vi "Evaporation LABView System.vi"() -> ()   [LabVIEW 2018]
uses:
  <vilib>/Utility/file.llb/Read Delimited Spreadsheet (DBL).vi
  <vilib>/Instr/_visa.llb/VISA Configure Serial Port (Instr).vi
  <instrlib>/JULABO DeviceDriver/JULABO DeviceDriver.lvlib
panel:
  in  "Mixing Time":dbl caption="Mixing Time (HH:MM)" format="%<%H:%M>t"
  out "Update Time":string
  out "Torque [Ncm]":string
  in  "Cent. Duration (MM:SS)":dbl caption="Duration\n(MM:SS)" format="%<%M:%S>t"
  in  "Speed":dbl
  in  "Syrup °Bx by Manual RF":dbl format="%#.1f"
  in  "°Bx DM":dbl caption="Syrup + Additive \n°Bx by Manual RF" format="%#.1f"
  out "Boolean 32":bool
  in  "Mixing RPM":dbl
  out "Boolean 28":bool
  out "Theoretical 5 min. TS":dbl caption="5 min." format="%#.2g"
  out "Boolean 33":bool
  in  "Silverson Duration (MM:SS)":dbl caption="Duration (MM:SS)" format="%<%M:%S>t"
  in  "Speed RPM":dbl
  out "Seeding Julabo SS Temp. [°C]":dbl format="%#.2f"
  out "Seeding Julabo Glass Temp. [°C]":dbl format="%#.2f"
  out "Seeding RPM":dbl format="%#.2f"
  out "Seeding Kss":dbl format="%#.2f"
  out "Seeding Temp. [°C]":dbl format="%#.1f"
  out "Seeding °Bx":dbl format="%#.2f"
  in  "Comments":string
  in  "Loading Delay":timestamp caption="Loading Delay (HH:MM)" format="%<%H:%M>T"
  in  "Additives":string
  in  "Percentage [%]":dbl format="%#_2g"
  in  "pH":dbl format="%#.2g"
  in  "Temp. [°C]":dbl format="%#.2g"
  in  "Sugar Source":string(combo)
  out "Boolean 23":bool
  out "Elapsed Time":dbl format="%.1f"
  out "Seed Time":timestamp format="%<%H:%M:%S>T"
  out "Total Solids (TS)":dbl format="%#.1g"
  in  "Config Tab":T1(tab)
  in  "Condensate Balance":refnum<visa-resource-name>
  in  "Refractometer":refnum<visa-resource-name>
  in  "Vacuubrand Pump":refnum<visa-resource-name>
  in  "Hei-Torque Stirrer":refnum<visa-resource-name>
  in  "Julabo Glass":refnum<visa-resource-name>="COM3"
  in  "Julabo Stainless Steel":refnum<visa-resource-name>="COM3"
  in  "Peristaltic Balance":refnum<visa-resource-name>
  in  "Peristaltic Pump":refnum<visa-resource-name>
  in  "Vacuubrand Pump":bool
  in  "Refractometer":bool
  in  "Condensate Balance":bool
  in  "Julabo Glass":bool
  in  "Hei-Torque Stirrer":bool
  in  "Peristaltic Balance":bool
  in  "Peristaltic Pump":bool
  out "Peristaltic Pump Restart":bool
  out "Hei-Torque Stirrer Restart":bool
  out "Refractometer Restart":bool
  out "Vacuubrand Pump Restart":bool
  out "Condensate Balance Restart":bool
  out "Peristaltic Balance Restart":bool
  out "Julabo Glass Restart":bool
  out "Julabo SS Restart":bool
  in  "Julabo Stainless Steel":bool
  in  "Stop Program":bool
  in  "Start/Stop\nRecording":bool
  out "Process Start":i32
  in  "Experiment Type":string(combo)
  in  "Operator Name":string
  in  "Experiment Name":string
  in  "Time Interval":dbl caption="Time Interval (MM:SS)" format="%<%M:%S>t"
  out "1 min. TS":dbl caption="1 min." format="%#.2g"
  in  "Graphs Tab":T2(tab)
  out "Supersaturation (Kss)":dbl format="%#.2g"
  out "Supersaturation Graph (Kss)":dbl(graph)
  out "Torque [Ncm]":string
  out "Torque Graph":dbl(graph)
  out "Process 2":dbl(graph)
  out "Process":dbl caption="Evaporation Rate [gr/min.]" format="%#.2g"
  out "TS-Mass Graph":cluster{dbl[], dbl[]}(graph) caption="Tank's Solution Weight [gr] vs. Total Solids [%]"
  out "dTS&dBX Graph":cluster{dbl, "Value":dbl}(graph) caption="dTS & dBX Change Rate [gr/min.]"
  in  "Seeds Added":bool
  in  "Add Seeds":bool
  in  "Method":string(combo)
  in  "Seed Type":string
  in  "Amount [gr]":dbl
  in  "Size (um)":string
  out "Theoretical Addition Rate [gr/min]":dbl format="%#.2g"
  in  "Add Syrup":bool
  in  "Syrup Addition [gr]":dbl(slide) scale=0.0..12500.0
  in  "Yield [%]":dbl
  in  "Emptying 2nd\nCycle [gr]":dbl
  in  "Emptying 1st\nCycle [gr]":dbl
  in  "Feed 2nd Cycle [gr]":dbl
  in  "Feed 1st Cycle [gr]":dbl
  out "Boolean 31":bool
  out "Boolean 27":bool
  out "Boolean 30":bool
  out "Boolean 29":bool
  out "Boolean":bool
  out "Peristaltic Pump":bool
  out "RF Pipe":bool
  out "Boolean 19":bool
  in  "Loading 2nd\nCycle [gr]":dbl
  in  "Loading 1st\nCycle [gr]":dbl
  out "Boolean 22":bool
  out "Boolean 2":bool
  out "Vacuubrand Pump":bool
  out "Temp. [°C]":dbl format="%#.2f"
  out "Temp. [°C] by PT100":dbl format="%#.2f"
  out "Tank's Height [cm]":dbl format="%#.1f"
  out "Tank's\nHeight [cm]":dbl(slide) scale=0.0..70.0
  out "Condensate Weight [gr]":dbl format="%#.1f"
  out "Torque [Ncm]":string
  out "Temp. [°C] by RF":dbl format="%#.1f"
  out "°Bx":dbl format="%#.2f"
  out "Syrup Added [gr]":dbl format="%#.1f"
  out "Addition Rate 1 min. [gr/min]":dbl format="%#.2g"
  in  "Dry Substance [%]":dbl
  in  "Purity (0.92-1.0)":dbl
  out "Total Amount Added [gr]":dbl
  in  "Speed RPM":dbl
  in  "Start/Stop":bool
  out "Syrup Added [gr]":dbl(slide) scale=0.0..12500.0
  out "Dry Substance [%]":dbl(slide) scale=0.0..100.0 scale format="%.2f"
  out "1 min. BX":dbl caption="1 min." format="%#.2g"
  out "Colors4":cluster{u32, u32}[](array[cluster])=[{12369084, 12369084}, {255, 255}, {7995525, 7995525}, {7995525, 7995525}]
  out "Interpolated Data":dbl[][](array[numeric])
  out "Table Value":dbl
  out "Actual Saturation (Kact)":dbl format="%#.2g"
  out "Saturation (Ks)":dbl format="%#.2g"
  in  "°Bx In-Line":dbl caption="°Bx by In-Line RF" format="%#.2f"
  in  "Purity (0.92-1.0)":dbl
  out "5 min.":dbl format="%#.2g"
  out "20 min.":dbl format="%#.2g"
  out "Amount of Dry Substance\n[gr]":dbl
  out "Amount of Sugar [gr]":dbl
  out "Dry Substance [%]":dbl(slide) scale=0.0..100.0 scale format="%.2f"
  out "Sugar [%]":dbl(slide) scale=0.0..100.0 scale format="%.2f"
  out "Refractive Index":dbl format="%#.5f"
  out "Temp. [°C]":dbl format="%#.1f"
  out "°Bx":dbl format="%#.2f"
  out "Stirrer Paddle":bool
  out "Tank's Solution\nWeight [gr]":dbl(slide) scale=0.0..12500.0
  out "Boolean 17":bool
  out "Boolean 16":bool
  out "Boolean 15":bool
  out "Boolean 14":bool
  out "Boolean 13":bool
  out "Boolean 12":bool
  out "Boolean 11":bool
  out "Boolean 10":bool
  out "Condensate Weight [gr]":dbl(slide) scale=0.0..3500.0
  out "Boolean 9":bool
  out "Boolean 8":bool
  out "Boolean 7":bool
  out "Boolean 6":bool
  out "Boolean 5":bool
  out "Boolean 4":bool
  out "Boolean 3":bool
  out "Boolean 1":bool
  out "Internal Temp.":dbl(slide) scale=0.0..150.0
  in  "Start/\nStop":bool
  in  "Set Temp. [°C]":dbl format="%.2f"
  out "Internal Temp.":dbl(slide) scale=0.0..150.0
  in  "Start/\nStop":bool
  in  "Set Temp. [°C]":dbl format="%.2f"
  in  "Set Speed RPM":dbl
  in  "Set Vacuum [mbar]":dbl
  in  "Start/Stop":bool
  in  "Vent":bool
  out "Current\nPressure\n[mbar]":dbl(knob) scale=1050.0..50.0
  out "Boolean 20":bool
  out "Boolean 18":bool
  out "Boolean 21":bool
  out "Boolean 26":bool
  out "Boolean 25":bool
  out "Pipe Delay":dbl
  out "Boolean 24":bool
  # "Amounts Added"
  # "Seeding"
  # "Hei-Torque Stirrer"
  # "Condensate\nBalance"
  # "PT100 Sensor"
  # "Julabo Glass"
  # "Refractometer"
  # "Syrup Loading"
  # "Julabo Stainless Steel"
  # "Silverson Mixer"
  # "Centrifugation"
  # "Syrup Preparation Station"
  # "Peristaltic Pump"
  # "Fluidized Bed Dryer"
  # "Values Updated Every 5 min."
  # "Please make sure\nthat all the\ncentrifugation and\nfluidized bed\ndryer values are\nupdated before\npressing \"Stop\nProgram\" or\n\"Stop Recording\"!"
  # "Evaporation\nRate [gr/min]"
  # "BX Change\nRate [gr/min]"
  # "TS Change\nRate [gr/min]"
  # "Theoretical TS Change\nRate [gr/min]"
  # "Peristaltic Balance"
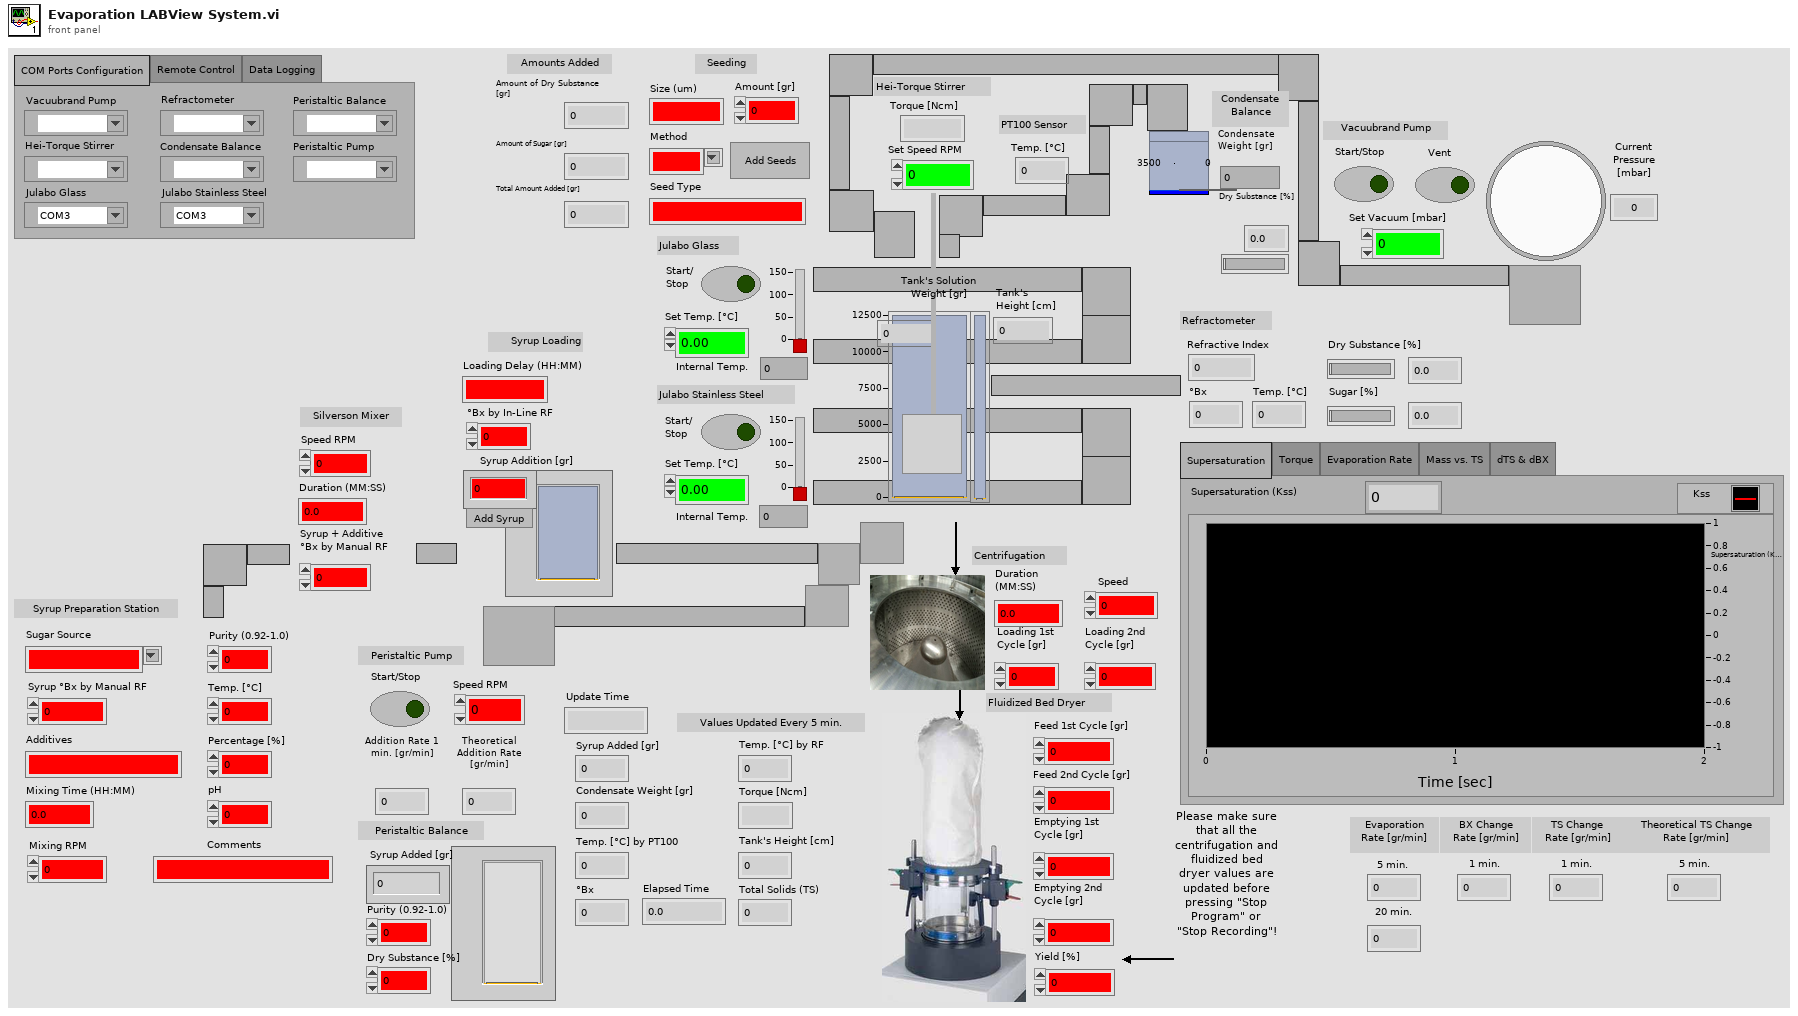
[diagram p1: front panel]
types:
  T1 = enum32{"COM Ports Configuration", "Remote Control", "Data Logging"}
  T2 = enum32{"Supersaturation", "Torque", "Evaporation Rate", "Mass vs. TS", "dTS & dBX"}
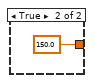
[diagram p5: hidden frame]
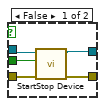
[diagram p6: hidden frame]
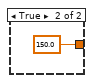
[diagram p10: hidden frame]
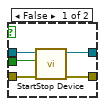
[diagram p11: hidden frame]
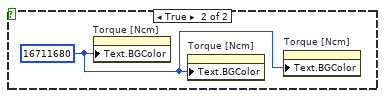
[diagram p16: hidden frame]
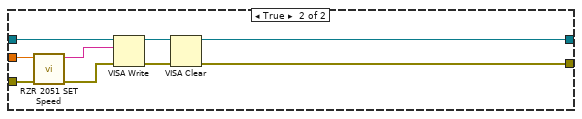
[diagram p17: hidden frame]
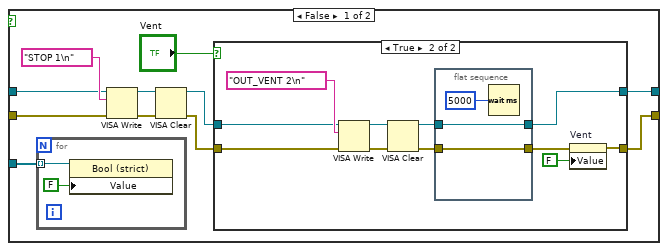
[diagram p20: hidden frame]
diagram:
  n1 = while {
    stop <- w5 stop-if-true
    n2 = property on="Stop Program" class="Bool (strict)"() -> ("Value"=w5:bool)  [unwired: 2 in, 2 out]
    n3 = Wait (ms)(milliseconds to wait=u32 1000) -> ()  [unwired: 1 out]
    n4 = case shown="True" "Vacuubrand Pump" {
      frame False {
      }
      frame True {
        n5 = flat-sequence {
          tunnel: [w26] -> w16
          tunnel: [w25] -> w15
          tunnel: w16 -> [w58]
          tunnel: w15 -> [w57]
          tunnel: [w44] -> w14
          tunnel: [w43] -> w13
          tunnel: [w31] -> w10
          tunnel: w14 -> [w68]
          tunnel: w13 -> [w67]
          tunnel: [w66] -> w12
          tunnel: [w65] -> w11
          tunnel: w10 -> [w64]
          tunnel: [w63] -> w9
          tunnel: w12 -> [w171]
          tunnel: w11 -> [w170]
          tunnel: w9 -> [w160]
          tunnel: [w159] -> w8
          tunnel: [w158] -> w7
          tunnel: w8 -> [w184]
          tunnel: w7 -> [w183]
          frame #0 {
            w27 = u16 10 items=["1.0"=10, "1.5"=15, "2.0"=20] ("stop bits (10: 1 bit)")
            n6 = property on="Start/Stop" class="Bool (strict)"("Value"=FALSE ("PressON/OFF")) -> ()  [unwired: 2 in, 2 out]
            n7 = property on="Vent" class="Bool (strict)"("Value"=FALSE ("PressON/OFF")) -> ()  [unwired: 2 in, 2 out]
            n8 = call-poly "VISA Configure Serial Port"("VISA resource name"="Vacuubrand Pump", "baud rate (9600)"=u32 19200, "data bits (8)"=u16 8, "parity (0:none)"=enum16{"None", "Odd", "Even", "Mark", "Space"}."None", "stop bits (10: 1 bit)"=w27, "flow control (0:none)"=enum16{"None", "XON/XOFF", "RTS/CTS", "DTR/DSR"}."RTS/CTS" ("parity (0:none)")) -> ("VISA resource name out"=w26:refnum<visa-resource-name>, "error out"=w25:errorcluster)  [unwired: 8 in]
            n9 = property on="Set Vacuum [mbar]" class="DigNum (strict)"("Value"=1050.0, "NumText.BGColor"=u32 16711680 ("Numeric Text.Text Colors:BG Color")) -> ()  [unwired: 2 in, 2 out]
            n10 = property on="Current\nPressure\n[mbar]" class="Knob (strict)"("Value"=1050.0 ("Current Pressure [mbar]")) -> ()  [unwired: 2 in, 2 out]
            n11 = property on="Vacuubrand Pump Restart" class="Bool (strict)"("Value"=FALSE ("Vacuubrand Pump Restart")) -> ()  [unwired: 2 in, 2 out]
          }
          frame #1 {
            n12 = control-ref of="Boolean 4"() -> (w37:refnum<vi>)
            n13 = control-ref of="Boolean 3"() -> (w36:refnum<vi>)
            n14 = control-ref of="Boolean 2"() -> (w35:refnum<vi>)
            n15 = control-ref of="Boolean 1"() -> (w34:refnum<vi>)
            n16 = control-ref of="Vacuubrand Pump"() -> (w33:refnum<vi>)
            n17 = VISA Write(VISA resource name=w58, write buffer="REMOTE 1\n" ("Command"), error in (no error)=w57) -> (VISA resource name out=w56:refnum<visa-resource-name>, error out=w55:errorcluster)  [unwired: 1 out]
            n18 = control-ref of="Boolean 9"() -> (w38:refnum<vi>)
            n19 = control-ref of="Boolean 8"() -> (w39:refnum<vi>)
            n20 = control-ref of="Boolean 7"() -> (w40:refnum<vi>)
            n21 = control-ref of="Boolean 6"() -> (w41:refnum<vi>)
            n22 = control-ref of="Boolean 5"() -> (w42:refnum<vi>)
            n23 = VISA Clear(VISA resource name=w56, error in (no error)=w55) -> (VISA resource name out=w54:refnum<visa-resource-name>, error out=w51:errorcluster)
            n24 = VISA Write(VISA resource name=w54, write buffer="CVC 3\n" ("Command"), error in (no error)=w51) -> (VISA resource name out=w53:refnum<visa-resource-name>, error out=w52:errorcluster)  [unwired: 1 out]
            n25 = Build Array(w37, w36, w35, w34, w33, w38, w39, w40, w41, w42) -> (w32:refnum<vi>[])
            n26 = VISA Clear(VISA resource name=w53, error in (no error)=w52) -> (VISA resource name out=w48:refnum<visa-resource-name>, error out=w47:errorcluster)
            n27 = for {
              tunnel: w32 -> [w62] mode=indexing
              tunnel: [w60] -> w31 mode=indexing
              n28 = property class="Bool (strict)"(reference=w62, "Value"=FALSE) -> (reference out=w60:refnum<vi>)  [unwired: 1 in, 1 out]
            }
            n29 = VISA Write(VISA resource name=w48, write buffer="OUT_MODE 2\n" ("Command"), error in (no error)=w47) -> (VISA resource name out=w45:refnum<visa-resource-name>, error out=w46:errorcluster)  [unwired: 1 out]
            n30 = VISA Clear(VISA resource name=w45, error in (no error)=w46) -> (VISA resource name out=w44:refnum<visa-resource-name>, error out=w43:errorcluster)
          }
          frame #2 {
            n31 = while {
              tunnel: w68 -> [w100]
              tunnel: w67 -> [w99]
              shift-right: [w78] -> _
              shift-left: _ -> [w80]
              tunnel: [w94] -> w66
              tunnel: [w93] -> w65
              tunnel: w64 -> [w70]
              tunnel: [w70] -> w63
              stop <- w77 stop-if-true
              n32 = Less?(x="Set Vacuum [mbar]", y=90.0) -> (x < y?=w82:bool)
              n33 = Wait (ms)(milliseconds to wait=u32 1000) -> ()  [unwired: 1 out]
              n34 = case shown="True" w82 {
                tunnel: [w102 90.0] -> w78
                tunnel: "Set Vacuum [mbar]" -> [w102 _]
                frame False {
                }
                frame True {
                  n35 = property on="Set Vacuum [mbar]" class="DigNum (strict)"("Value"=90.0) -> ()  [unwired: 2 in, 2 out]
                }
              }
              n36 = property on="Vacuubrand Pump" class="Bool (strict)"() -> ("Value"=w71:bool)  [unwired: 2 in, 2 out]
              n37 = property on="Stop Program" class="Bool (strict)"() -> ("Value"=w72:bool)  [unwired: 2 in, 2 out]
              n38 = Not(x=w71) -> (.not. x?=w69:bool)
              n39 = Or(x=w69, y=w72) -> (x .or. y?=w77:bool)
              n40 = Not Equal?(x=w78, y=w80) -> (x != y?=w79:bool)
              n41 = case shown="True" w79 {
                tunnel: w78 -> [_ w150]
                tunnel: w99 -> [w147 w155]
                tunnel: w100 -> [w148 w154]
                tunnel: [w148 w153] -> w98
                tunnel: [w147 w152] -> w97
                frame False {
                }
                frame True {
                  n42 = property on="Set Vacuum [mbar]" class="DigNum (strict)"("NumText.BGColor"=u32 65280 ("Numeric Text.Text Colors:BG Color")) -> ()  [unwired: 2 in, 2 out]
                  n43 = call "Crystallization Vaccubrand Pump Set Vacuum.vi"("Vacuum [mbar]"=w150) -> ("DATA OUT"=w151:string)  [unwired: 10 in]
                  n44 = VISA Write(VISA resource name=w154, write buffer=w151, error in (no error)=w155) -> (VISA resource name out=w156:refnum<visa-resource-name>, error out=w157:errorcluster)  [unwired: 1 out]
                  n45 = VISA Clear(VISA resource name=w156, error in (no error)=w157) -> (VISA resource name out=w153:refnum<visa-resource-name>, error out=w152:errorcluster)
                }
              }
              n46 = case shown="True" "Start/Stop" {
                tunnel: w98 -> [w115 w139]
                tunnel: w97 -> [w114 w138]
                tunnel: [w113 w141] -> w96
                tunnel: [w112 w140] -> w95
                tunnel: w70 -> [w108 w137]
                frame False {
                  n47 = for {
                    tunnel: w108 -> [w120] mode=indexing
                    n48 = property class="Bool (strict)"(reference=w120, "Value"=FALSE) -> ()  [unwired: 1 in, 2 out]
                  }
                  n49 = VISA Write(VISA resource name=w115, write buffer="STOP 1\n" ("Command"), error in (no error)=w114) -> (VISA resource name out=w118:refnum<visa-resource-name>, error out=w117:errorcluster)  [unwired: 1 out]
                  n50 = VISA Clear(VISA resource name=w118, error in (no error)=w117) -> (VISA resource name out=w111:refnum<visa-resource-name>, error out=w110:errorcluster)
                  n51 = case shown="True" "Vent" {
                    tunnel: [w122 w128] -> w113
                    tunnel: [w121 w124] -> w112
                    tunnel: w111 -> [w122 w127]
                    tunnel: w110 -> [w121 w126]
                    frame False {
                    }
                    frame True {
                      n52 = VISA Write(VISA resource name=w127, write buffer="OUT_VENT 2\n" ("Command"), error in (no error)=w126) -> (VISA resource name out=w130:refnum<visa-resource-name>, error out=w131:errorcluster)  [unwired: 1 out]
                      n53 = VISA Clear(VISA resource name=w130, error in (no error)=w131) -> (VISA resource name out=w133:refnum<visa-resource-name>, error out=w132:errorcluster)
                      n54 = flat-sequence {
                        tunnel: w133 -> [w136]
                        tunnel: w132 -> [w135]
                        tunnel: [w136] -> w128
                        tunnel: [w135] -> w123
                        frame #0 {
                          n55 = Wait (ms)(milliseconds to wait=u32 5000) -> ()  [unwired: 1 out]
                        }
                      }
                      n56 = property on="Vent" class="Bool (strict)"(error in=w123, "Value"=FALSE ("PressON/OFF")) -> (error out=w124:errorcluster)  [unwired: 1 in, 1 out]
                    }
                  }
                }
                frame True {
                  n57 = for {
                    tunnel: w137 -> [w146] mode=indexing
                    n58 = property class="Bool (strict)"(reference=w146, "Value"=TRUE) -> ()  [unwired: 1 in, 2 out]
                  }
                  n59 = VISA Write(VISA resource name=w139, write buffer="START\n" ("Command"), error in (no error)=w138) -> (VISA resource name out=w144:refnum<visa-resource-name>, error out=w143:errorcluster)  [unwired: 1 out]
                  n60 = VISA Clear(VISA resource name=w144, error in (no error)=w143) -> (VISA resource name out=w141:refnum<visa-resource-name>, error out=w140:errorcluster)
                }
              }
              n61 = VISA Write(VISA resource name=w96, write buffer="IN_PV_1\n" ("Command"), error in (no error)=w95) -> (VISA resource name out=w92:refnum<visa-resource-name>, error out=w91:errorcluster)  [unwired: 1 out]
              n62 = flat-sequence {
                tunnel: w92 -> [w107]
                tunnel: w91 -> [w106]
                tunnel: [w107] -> w90
                tunnel: [w106] -> w89
                frame #0 {
                  n63 = Wait (ms)(milliseconds to wait=u32 500) -> ()  [unwired: 1 out]
                }
              }
              n64 = property class="Instr"(reference=w90, error in=w89) -> (reference out=w88:refnum<visa-resource-name>, error out=w87:errorcluster, "Serial Settings:Number of Bytes at Serial Port"=w86:u32)
              n65 = VISA Read(VISA resource name=w88, byte count=w86, error in (no error)=w87) -> (VISA resource name out=w94:refnum<visa-resource-name>, read buffer=w83:string, error out=w93:errorcluster)  [unwired: 1 out]
              n66 = String Subset(string=w83, length (rest)=4) -> (substring=w74:string)  [unwired: 1 in]
              n67 = Fract/Exp String To Number(string=w74) -> (number=→"Current\nPressure\n[mbar]":dbl)  [unwired: 3 in, 1 out]
            }
          }
          frame #3 {
            n68 = for {
              tunnel: w160 -> [w179] mode=indexing
              n69 = property class="Bool (strict)"(reference=w179, "Value"=FALSE) -> ()  [unwired: 1 in, 2 out]
            }
            n70 = VISA Write(VISA resource name=w171, write buffer="STOP 1\n" ("Command"), error in (no error)=w170) -> (VISA resource name out=w173:refnum<visa-resource-name>, error out=w174:errorcluster)  [unwired: 1 out]
            n71 = VISA Clear(VISA resource name=w173, error in (no error)=w174) -> (VISA resource name out=w168:refnum<visa-resource-name>, error out=w166:errorcluster)
            n72 = VISA Write(VISA resource name=w168, write buffer="OUT_VENT 2\n" ("Command"), error in (no error)=w166) -> (VISA resource name out=w167:refnum<visa-resource-name>, error out=w165:errorcluster)  [unwired: 1 out]
            n73 = VISA Clear(VISA resource name=w167, error in (no error)=w165) -> (VISA resource name out=w164:refnum<visa-resource-name>, error out=w163:errorcluster)
            n74 = flat-sequence {
              tunnel: w164 -> [w182]
              tunnel: w163 -> [w181]
              tunnel: [w182] -> w162
              tunnel: [w181] -> w161
              frame #0 {
                n75 = Wait (ms)(milliseconds to wait=u32 5000) -> ()  [unwired: 1 out]
              }
            }
            n76 = VISA Write(VISA resource name=w162, write buffer="REMOTE 0\n" ("Command"), error in (no error)=w161) -> (VISA resource name out=w176:refnum<visa-resource-name>, error out=w177:errorcluster)  [unwired: 1 out]
            n77 = VISA Clear(VISA resource name=w176, error in (no error)=w177) -> (VISA resource name out=w159:refnum<visa-resource-name>, error out=w158:errorcluster)
          }
          frame #4 {
            n78 = VISA Close(VISA resource name=w184, error in (no error)=w183) -> (error out=w185:errorcluster)
            n79 = call <vilib>:"Simple Error Handler.vi"("error in (no error)"=w185) -> ()  [unwired: 1 in, 8 out]
          }
          frame #5 {
            "Vacuubrand Pump Restart" <- TRUE ("Vacuubrand Pump Restart")
          }
        }
      }
    }
  }
  n80 = while {
    stop <- w187 stop-if-true
    n81 = property on="Stop Program" class="Bool (strict)"() -> ("Value"=w187:bool)  [unwired: 2 in, 2 out]
    n82 = Wait (ms)(milliseconds to wait=u32 1000) -> ()  [unwired: 1 out]
    n83 = case shown="True" "Hei-Torque Stirrer" {
      frame False {
      }
      frame True {
        n84 = flat-sequence {
          tunnel: [w206] -> w198
          tunnel: [w205] -> w199
          tunnel: w199 -> [w213]
          tunnel: w198 -> [w212]
          tunnel: [w215] -> w197
          tunnel: [w214] -> w196
          tunnel: [w211] -> w195
          tunnel: w197 -> [w223]
          tunnel: w196 -> [w220]
          tunnel: w195 -> [w224]
          tunnel: [w225] -> w194
          tunnel: [w222] -> w193
          tunnel: [w221] -> w192
          tunnel: w194 -> [w258]
          tunnel: w193 -> [w260]
          tunnel: w192 -> [w259]
          tunnel: [w262] -> w191
          tunnel: [w261] -> w190
          tunnel: w191 -> [w300]
          tunnel: w190 -> [w301]
          frame #0 {
            w207 = u16 10 items=["1.0"=10, "1.5"=15, "2.0"=20] ("stop bits (10: 1 bit)")
            n85 = property on="Set Speed RPM" class="DigNum (strict)"("Value"=0.0, "NumText.BGColor"=u32 16711680 ("Numeric Text.Text Colors:BG Color")) -> ()  [unwired: 2 in, 2 out]
            n86 = call-poly "VISA Configure Serial Port"("VISA resource name"="Hei-Torque Stirrer", "baud rate (9600)"=u32 9600, "data bits (8)"=u16 8, "parity (0:none)"=enum16{"None", "Odd", "Even", "Mark", "Space"}."None", "stop bits (10: 1 bit)"=w207) -> ("VISA resource name out"=w206:refnum<visa-resource-name>, "error out"=w205:errorcluster)  [unwired: 9 in]
            n87 = property on="Hei-Torque Stirrer Restart" class="Bool (strict)"("Value"=FALSE ("Hei-Torque Stirrer Restart")) -> ()  [unwired: 2 in, 2 out]
            "Stirrer Paddle" <- FALSE ("Stirrer Paddle")
          }
          frame #1 {
            w211 = 0.0 ("Speed RPM")
            # "Start communication to the stirrer"
            n88 = call "RZR 2051 SET Speed.vi"("ERROR IN"=w213, "Speed RPM"=w211) -> ("ERROR OUT"=w217:errorcluster, "DATA OUT"=w216:string)  [unwired: 8 in]
            n89 = VISA Write(VISA resource name=w212, write buffer=w216, error in (no error)=w217) -> (VISA resource name out=w219:refnum<visa-resource-name>, error out=w218:errorcluster)  [unwired: 1 out]
            n90 = VISA Clear(VISA resource name=w219, error in (no error)=w218) -> (VISA resource name out=w214:refnum<visa-resource-name>, error out=w215:errorcluster)
          }
          frame #2 {
            n91 = while {
              tunnel: w223 -> [w240]
              tunnel: [w239] -> w222
              tunnel: [w238] -> w221
              tunnel: w220 -> [w237]
              shift-right: [w233] -> w225
              shift-left: w224 -> [w241]
              stop <- w226 stop-if-true
              n92 = Greater?(x="Set Speed RPM", y=500.0) -> (0:w234:bool)
              n93 = case shown="True" w234 {
                tunnel: [w242 500.0] -> w233
                tunnel: "Set Speed RPM" -> [w242 _]
                frame False {
                }
                frame True {
                  n94 = property on="Set Speed RPM" class="DigNum (strict)"("Value"=500.0) -> ()  [unwired: 2 in, 2 out]
                }
              }
              n95 = Wait (ms)(milliseconds to wait=u32 500) -> ()  [unwired: 1 out]
              n96 = Not Equal?(x=w233, y=w241) -> (x != y?=w227:bool)
              n97 = case shown="True" w227 {
                tunnel: w240 -> [w245 w251]
                tunnel: [w245 w250] -> w239
                tunnel: [w246 w249] -> w238
                tunnel: w237 -> [w246 w248]
                tunnel: w233 -> [_ w247]
                frame False {
                }
                frame True {
                  n98 = call "RZR 2051 SET Speed.vi"("ERROR IN"=w251, "Speed RPM"=w247) -> ("ERROR OUT"=w254:errorcluster, "DATA OUT"=w252:string)  [unwired: 8 in]
                  n99 = VISA Write(VISA resource name=w248, write buffer=w252, error in (no error)=w254) -> (VISA resource name out=w255:refnum<visa-resource-name>, error out=w253:errorcluster)  [unwired: 1 out]
                  n100 = VISA Clear(VISA resource name=w255, error in (no error)=w253) -> (VISA resource name out=w249:refnum<visa-resource-name>, error out=w250:errorcluster)
                }
              }
              n101 = property on="Hei-Torque Stirrer" class="Bool (strict)"() -> ("Value"=w230:bool)  [unwired: 2 in, 2 out]
              n102 = property on="Stop Program" class="Bool (strict)"() -> ("Value"=w231:bool)  [unwired: 2 in, 2 out]
              n103 = Not(x=w230) -> (.not. x?=w229:bool)
              n104 = Or(x=w229, y=w231) -> (x .or. y?=w228:bool)
              n105 = Or(x=w227, y=w228) -> (x .or. y?=w226:bool)
            }
          }
          frame #3 {
            n106 = while {
              tunnel: w260 -> [w276]
              tunnel: w259 -> [w271]
              shift-right: [w268] -> _
              shift-left: w258 -> [w274]
              tunnel: [w273] -> w262
              tunnel: [w272] -> w261
              stop <- w267 stop-if-true
              n107 = property on="Set Speed RPM" class="DigNum (strict)"() -> ("Value"=w265:dbl)  [unwired: 2 in, 2 out]
              n108 = property on="Hei-Torque Stirrer" class="Bool (strict)"() -> ("Value"=w264:bool)  [unwired: 2 in, 2 out]
              n109 = property on="Stop Program" class="Bool (strict)"() -> ("Value"=w266:bool)  [unwired: 2 in, 2 out]
              n110 = Not(x=w264) -> (.not. x?=w263:bool)
              n111 = Greater?(x=w265, y=500.0) -> (0:w270:bool)
              n112 = case shown="True" w270 {
                tunnel: [w278 500.0] -> w268
                tunnel: w265 -> [w278 _]
                frame False {
                }
                frame True {
                  n113 = property on="Set Speed RPM" class="DigNum (strict)"("Value"=500.0) -> ()  [unwired: 2 in, 2 out]
                }
              }
              n114 = Or(x=w263, y=w266) -> (x .or. y?=w267:bool)
              n115 = Wait (ms)(milliseconds to wait=u32 1000) -> ()  [unwired: 1 out]
              n116 = Not Equal?(x=w268, y=w274) -> (x != y?=w275:bool)
              n117 = case shown="False" w275 {
                tunnel: w276 -> [w287 w298]
                tunnel: w271 -> [w285 w297]
                tunnel: [w286 w292] -> w273
                tunnel: [w285 w291] -> w272
                tunnel: w268 -> [_ w290]
                frame False {
                  n118 = call "RZR 2051 Read TORQUE.vi"("ERROR IN"=w287, "COM PORT IN"=w285) -> ("ERROR OUT"=w286:errorcluster, "DATA OUT"=w282:dbl, "STRING OUT"=→"Torque [Ncm]" →"Torque [Ncm]":string)  [unwired: 7 in]
                  "Torque Graph" <- w282
                  n119 = Greater Or Equal?(x=w282, y=50.0) -> (x >= y?=w283:bool)
                  n120 = case shown="False" w283 {
                    frame False {
                      w288 = u32 13816530
                      n121 = property on="Torque [Ncm]" class="Str"("Text.BGColor"=w288) -> ()  [unwired: 2 in, 2 out]
                      n122 = property on="Torque [Ncm]" class="Str"("Text.BGColor"=w288) -> ()  [unwired: 2 in, 2 out]
                      n123 = property on="Torque [Ncm]" class="Str"("Text.BGColor"=w288) -> ()  [unwired: 2 in, 2 out]
                    }
                    frame True {
                      w289 = u32 16711680 ("Numeric Text.Text Colors:BG Color")
                      n124 = property on="Torque [Ncm]" class="Str"("Text.BGColor"=w289) -> ()  [unwired: 2 in, 2 out]
                      n125 = property on="Torque [Ncm]" class="Str"("Text.BGColor"=w289) -> ()  [unwired: 2 in, 2 out]
                      n126 = property on="Torque [Ncm]" class="Str"("Text.BGColor"=w289) -> ()  [unwired: 2 in, 2 out]
                    }
                  }
                }
                frame True {
                  n127 = call "RZR 2051 SET Speed.vi"("ERROR IN"=w298, "Speed RPM"=w290) -> ("ERROR OUT"=w295:errorcluster, "DATA OUT"=w293:string)  [unwired: 8 in]
                  n128 = VISA Write(VISA resource name=w297, write buffer=w293, error in (no error)=w295) -> (VISA resource name out=w296:refnum<visa-resource-name>, error out=w294:errorcluster)  [unwired: 1 out]
                  n129 = VISA Clear(VISA resource name=w296, error in (no error)=w294) -> (VISA resource name out=w291:refnum<visa-resource-name>, error out=w292:errorcluster)
                }
              }
            }
            n130 = property on="Stirrer Paddle" class="Bool (strict)"("Value"=TRUE ("Stirrer Paddle")) -> ()  [unwired: 2 in, 2 out]
            n131 = property on="Set Speed RPM" class="DigNum (strict)"("NumText.BGColor"=u32 65280 ("Numeric Text.Text Colors:BG Color")) -> ()  [unwired: 2 in, 2 out]
          }
          frame #4 {
            n132 = call <instrlib>:"RZR 2051 STOP Communication.vi"("Error IN"=w300, "COM Port"=w301) -> ("Error OUT"=w302:errorcluster)  [unwired: 9 in]
            n133 = property on="Stirrer Paddle" class="Bool (strict)"("Value"=FALSE ("Stirrer Paddle")) -> ()  [unwired: 2 in, 2 out]
            n134 = call <vilib>:"General Error Handler.vi"("error in (no error)"=w302) -> ()  [unwired: 10 in, 5 out]
          }
          frame #5 {
            "Hei-Torque Stirrer Restart" <- TRUE ("Hei-Torque Stirrer Restart")
          }
        }
      }
    }
  }
  n135 = while {
    stop <- w304 stop-if-true
    n136 = property on="Stop Program" class="Bool (strict)"() -> ("Value"=w304:bool)  [unwired: 2 in, 2 out]
    n137 = Wait (ms)(milliseconds to wait=u32 1000) -> ()  [unwired: 1 out]
    n138 = case shown="True" "Peristaltic Pump" {
      frame False {
      }
      frame True {
        n139 = flat-sequence {
          tunnel: [w327] -> w312
          tunnel: [w326] -> w311
          tunnel: [w321] -> w310
          tunnel: w312 -> [w342]
          tunnel: w311 -> [w341]
          tunnel: w310 -> [w335]
          tunnel: [w340] -> w309
          tunnel: [w339] -> w308
          tunnel: [w336] -> w307
          tunnel: w309 -> [w403]
          tunnel: w308 -> [w402]
          tunnel: w307 -> [w405]
          frame #0 {
            w328 = u16 10 items=["1.0"=10, "1.5"=15, "2.0"=20] ("stop bits (10: 1 bit)")
            n140 = control-ref of="Peristaltic Pump"() -> (w319:refnum<vi>)
            n141 = control-ref of="Boolean 29"() -> (w320:refnum<vi>)
            n142 = control-ref of="Boolean 26"() -> (w318:refnum<vi>)
            n143 = control-ref of="Boolean 30"() -> (w317:refnum<vi>)
            n144 = control-ref of="Boolean"() -> (w316:refnum<vi>)
            n145 = Build Array(w319, w320, w318, w317, w316) -> (w322:refnum<vi>[])
            n146 = call-poly "VISA Configure Serial Port"("VISA resource name"="Peristaltic Pump", "baud rate (9600)"=u32 9600, "data bits (8)"=u16 8, "parity (0:none)"=enum16{"None", "Odd", "Even", "Mark", "Space"}."None", "stop bits (10: 1 bit)"=w328, "flow control (0:none)"=enum16{"None", "XON/XOFF", "RTS/CTS", "DTR/DSR"}."None" ("parity (0:none)")) -> ("VISA resource name out"=w327:refnum<visa-resource-name>, "error out"=w326:errorcluster)  [unwired: 8 in]
            n147 = for {
              tunnel: w322 -> [w334] mode=indexing
              tunnel: [w332] -> w321 mode=indexing
              n148 = property class="Bool (strict)"(reference=w334, "Value"=FALSE) -> (reference out=w332:refnum<vi>)  [unwired: 1 in, 1 out]
            }
            n149 = property on="Speed RPM" class="DigNum (strict)"("Value"=0.0 ("Speed RPM"), "NumText.BGColor"=u32 16711680 ("Numeric Text.Text Colors:BG Color")) -> ()  [unwired: 2 in, 2 out]
            n150 = property on="Peristaltic Pump Restart" class="Bool (strict)"("Value"=FALSE ("Peristaltic Pump Restart")) -> ()  [unwired: 2 in, 2 out]
            n151 = property on="Start/Stop" class="Bool (strict)"("Value"=FALSE ("Start/Stop")) -> ()  [unwired: 2 in, 2 out]
          }
          frame #1 {
            n152 = while {
              tunnel: w342 -> [w356]
              tunnel: w341 -> [w355]
              shift-right: [w354] -> _
              shift-left: 0.0 ("Speed RPM") -> [w358]
              tunnel: [w351] -> w340
              tunnel: [w350] -> w339
              shift-right: ["Start/Stop"] -> _
              shift-left: FALSE ("Start/Stop") -> [w352]
              tunnel: [w345] -> w336
              tunnel: w335 -> [w346]
              stop <- w363 stop-if-true
              n153 = property on="Peristaltic Pump" class="Bool (strict)"() -> ("Value"=w362:bool)  [unwired: 2 in, 2 out]
              n154 = Greater?(x="Speed RPM", y=120.0) -> (0:w360:bool)
              n155 = case shown="True" w360 {
                tunnel: "Speed RPM" -> [w399 _]
                tunnel: [w399 120.0 ("Speed RPM")] -> w354
                frame False {
                }
                frame True {
                  n156 = property on="Speed RPM" class="DigNum (strict)"("Value"=120.0 ("Speed RPM")) -> ()  [unwired: 2 in, 2 out]
                }
              }
              n157 = Not(x=w362) -> (.not. x?=w343:bool)
              n158 = property on="Stop Program" class="Bool (strict)"() -> ("Value"=w344:bool)  [unwired: 2 in, 2 out]
              n159 = Wait (ms)(milliseconds to wait=u32 1000) -> ()  [unwired: 1 out]
              n160 = Or(x=w343, y=w344) -> (x .or. y?=w363:bool)
              n161 = Not Equal?(x=w354, y=w358) -> (x != y?=w357:bool)
              n162 = case shown="True" w357 {
                tunnel: w356 -> [w389 w397]
                tunnel: w355 -> [w388 w396]
                tunnel: [w389 w394] -> w348
                tunnel: [w388 w393] -> w349
                tunnel: w354 -> [_ w391]
                frame False {
                }
                frame True {
                  n163 = call "Crystallization Peristaltic Pump Set Speed.vi"("Speed RPM"=w391) -> ("DATA OUT"=w392:string)  [unwired: 10 in]
                  n164 = property on="Speed RPM" class="DigNum (strict)"("NumText.BGColor"=u32 65280 ("Numeric Text.Text Colors:BG Color")) -> ()  [unwired: 2 in, 2 out]
                  n165 = VISA Write(VISA resource name=w397, write buffer=w392, error in (no error)=w396) -> (VISA resource name out=w398:refnum<visa-resource-name>, error out=w395:errorcluster)  [unwired: 1 out]
                  n166 = VISA Clear(VISA resource name=w398, error in (no error)=w395) -> (VISA resource name out=w394:refnum<visa-resource-name>, error out=w393:errorcluster)
                }
              }
              n167 = Not Equal?(x="Start/Stop", y=w352) -> (x != y?=w353:bool)
              n168 = case shown="True" w353 {
                tunnel: [w367 w375] -> w351
                tunnel: [w366 w374] -> w350
                tunnel: w349 -> [w366 w372]
                tunnel: w348 -> [w367 w373]
                tunnel: "Start/Stop" -> [_ w370]
                tunnel: w346 -> [w365 w369]
                tunnel: [w365 w368] -> w345
                frame False {
                }
                frame True {
                  n169 = case shown="True" w370 {
                    tunnel: w369 -> [w379 w384]
                    tunnel: [w378 w383] -> w368
                    frame False {
                      n170 = for {
                        tunnel: w379 -> [w382] mode=indexing
                        tunnel: [w380] -> w378 mode=indexing
                        n171 = property class="Bool (strict)"(reference=w382, "Value"=FALSE) -> (reference out=w380:refnum<vi>)  [unwired: 1 in, 1 out]
                      }
                    }
                    frame True {
                      n172 = for {
                        tunnel: w384 -> [w387] mode=indexing
                        tunnel: [w385] -> w383 mode=indexing
                        n173 = property class="Bool (strict)"(reference=w387, "Value"=TRUE) -> (reference out=w385:refnum<vi>)  [unwired: 1 in, 1 out]
                      }
                    }
                  }
                  n174 = VISA Write(VISA resource name=w373, write buffer="TA2!" ("Command"), error in (no error)=w372) -> (VISA resource name out=w377:refnum<visa-resource-name>, error out=w376:errorcluster)  [unwired: 1 out]
                  n175 = VISA Clear(VISA resource name=w377, error in (no error)=w376) -> (VISA resource name out=w375:refnum<visa-resource-name>, error out=w374:errorcluster)
                }
              }
            }
          }
          frame #2 {
            n176 = for {
              tunnel: w405 -> [w407] mode=indexing
              n177 = property class="Bool (strict)"(reference=w407, "Value"=FALSE) -> ()  [unwired: 1 in, 2 out]
            }
            n178 = VISA Close(VISA resource name=w403, error in (no error)=w402) -> (error out=w404:errorcluster)
            n179 = call <vilib>:"Simple Error Handler.vi"("error in (no error)"=w404) -> ()  [unwired: 1 in, 8 out]
          }
          frame #3 {
            "Peristaltic Pump Restart" <- TRUE ("Peristaltic Pump")
          }
        }
      }
    }
  }
  n180 = while {
    stop <- w410 stop-if-true
    n181 = property on="Stop Program" class="Bool (strict)"() -> ("Value"=w410:bool)  [unwired: 2 in, 2 out]
    n182 = Wait (ms)(milliseconds to wait=u32 1000) -> ()  [unwired: 1 out]
    n183 = case shown="True" "Refractometer" {
      frame False {
        n184 = property on="RF Pipe" class="Bool (strict)"("Value"=FALSE ("RF Pipe")) -> ()  [unwired: 2 in, 2 out]
      }
      frame True {
        n185 = flat-sequence {
          tunnel: [w420] -> w416
          tunnel: [w421] -> w415
          tunnel: w416 -> [w431]
          tunnel: w415 -> [w432]
          tunnel: [w430] -> w414
          tunnel: [w429] -> w413
          tunnel: w414 -> [w496]
          tunnel: w413 -> [w495]
          frame #0 {
            w423 = u16 10 items=["1.0"=10, "1.5"=15, "2.0"=20] ("stop bits (10: 1 bit)")
            n186 = property on="1 min. BX" class="DigNum (strict)"("Value"=0.0 ("1 min. BX")) -> ()  [unwired: 2 in, 2 out]
            n187 = property on="Refractometer Restart" class="Bool (strict)"("Value"=FALSE ("Refractometer Restart")) -> ()  [unwired: 2 in, 2 out]
            n188 = call-poly "VISA Configure Serial Port"("VISA resource name"="Refractometer", "baud rate (9600)"=u32 9600, "data bits (8)"=u16 8, "parity (0:none)"=enum16{"None", "Odd", "Even", "Mark", "Space"}."None", "stop bits (10: 1 bit)"=w423, "flow control (0:none)"=enum16{"None", "XON/XOFF", "RTS/CTS", "DTR/DSR"}."None" ("parity (0:none)")) -> ("VISA resource name out"=w421:refnum<visa-resource-name>, "error out"=w420:errorcluster)  [unwired: 8 in]
          }
          frame #1 {
            n189 = while {
              tunnel: w432 -> [w452]
              tunnel: [w455] -> w430
              tunnel: w431 -> [w451]
              tunnel: [w454] -> w429
              shift-right: [w434] -> _
              shift-left: dbl[] [] -> [w435]
              i -> [w436]
              stop <- w450 stop-if-true
              n190 = property on="Refractometer" class="Bool (strict)"() -> ("Value"=w444:bool)  [unwired: 2 in, 2 out]
              n191 = property class="Instr"(reference=w452, error in=w451) -> (reference out=w447:refnum<visa-resource-name>, error out=w446:errorcluster, "Serial Settings:Number of Bytes at Serial Port"=w445:u32)
              n192 = property on="Stop Program" class="Bool (strict)"() -> ("Value"=w443:bool)  [unwired: 2 in, 2 out]
              n193 = Not(x=w444) -> (.not. x?=w442:bool)
              n194 = Or(x=w442, y=w443) -> (x .or. y?=w450:bool)
              n195 = Greater?(x=w445, y=u32 38) -> (0:w449:bool)
              n196 = case shown="True" w449 {
                tunnel: [w467 w494] -> w455
                tunnel: [w465 w493] -> w454
                tunnel: w445 -> [w470 w484]
                tunnel: w447 -> [w468 w483]
                tunnel: w446 -> [w466 w482]
                frame False {
                  n197 = Greater?(x=w470, y=u32 0) -> (0:w469:bool)
                  n198 = case shown="True" w469 {
                    tunnel: w468 -> [w473 w477]
                    tunnel: [w473 w476] -> w467
                    tunnel: w466 -> [w472 w475]
                    tunnel: [w472 w474] -> w465
                    frame False {
                    }
                    frame True {
                      n199 = VISA Clear(VISA resource name=w477, error in (no error)=w475) -> (VISA resource name out=w476:refnum<visa-resource-name>, error out=w474:errorcluster)
                    }
                  }
                }
                frame True {
                  n200 = VISA Read(VISA resource name=w483, byte count=w484, error in (no error)=w482) -> (VISA resource name out=w494:refnum<visa-resource-name>, read buffer=w478:string, error out=w493:errorcluster)  [unwired: 1 out]
                  n201 = String Subset(string=w478, length (rest)=8) -> (substring=w491:string)  [unwired: 1 in]
                  n202 = String Subset(string=w478, offset (0)=12, length (rest)=4) -> (substring=w489:string)
                  n203 = Fract/Exp String To Number(string=w491) -> (number=→"Refractive Index":dbl)  [unwired: 3 in, 1 out]
                  n204 = Fract/Exp String To Number(string=w489) -> (number=→"Temp. [°C]":dbl)  [unwired: 3 in, 1 out]
                  n205 = String Subset(string=w478, offset (0)=22, length (rest)=5) -> (substring=w486:string)
                  n206 = Fract/Exp String To Number(string=w486) -> (number=→"°Bx":dbl)  [unwired: 3 in, 1 out]
                }
              }
              n207 = Wait (ms)(milliseconds to wait=u32 1000) -> ()  [unwired: 1 out]
              n208 = Add(x=w436, y=1) -> (x+y=w438:i32)
              n209 = Greater?(x=w438, y=59) -> (0:w437:bool)
              n210 = property on="°Bx" class="DigNum (strict)"() -> ("Value"=w433:dbl)  [unwired: 2 in, 2 out]
              n211 = Build Array(w433) -> (w441:dbl[])
              n212 = Insert Into Array(array=w435, index=w436, new element=w441) -> (w434:dbl[])
              n213 = case shown="True" w437 {
                tunnel: w434 -> [_ w460]
                tunnel: w436 -> [_ w459]
                frame False {
                }
                frame True {
                  n214 = Subtract(x=w459, y=59) -> (x-y=w464:i32)
                  n215 = Index Array(array=w460, index #1=w459, index #2=w464) -> (element #1=w461:dbl, element #2=w462:dbl)
                  n216 = property on="1 min. TS" class="DigNum (strict)"() -> ("Value"=w456:dbl)  [unwired: 2 in, 2 out]
                  n217 = Subtract(x=w461, y=w462) -> (x-y=w457:dbl)
                  "1 min. BX" <- w457
                  n218 = Bundle("Value"=w456, w457) -> (→"dTS&dBX Graph":cluster{"Value":dbl, dbl})  [unwired: 1 in]
                }
              }
            }
            "RF Pipe" <- TRUE ("Boolean 29")
          }
          frame #2 {
            n219 = VISA Close(VISA resource name=w496, error in (no error)=w495) -> (error out=w498:errorcluster)
            n220 = property on="RF Pipe" class="Bool (strict)"("Value"=FALSE ("RF Pipe")) -> ()  [unwired: 2 in, 2 out]
            n221 = call <vilib>:"Simple Error Handler.vi"("error in (no error)"=w498) -> ()  [unwired: 1 in, 8 out]
          }
          frame #3 {
            "Refractometer Restart" <- TRUE ("Refractometer Restart")
          }
        }
      }
    }
  }
  n222 = while {
    stop <- w502 stop-if-true
    n223 = property on="Stop Program" class="Bool (strict)"() -> ("Value"=w502:bool)  [unwired: 2 in, 2 out]
    n224 = Wait (ms)(milliseconds to wait=u32 200) -> ()  [unwired: 1 out]
    n225 = case shown="True" "Start/Stop\nRecording" {
      frame False {
      }
      frame True {
        n226 = flat-sequence {
          tunnel: [w531] -> w508
          tunnel: [w532] -> w507
          tunnel: [w543] -> w510
          tunnel: [w544] -> w509
          tunnel: w507 -> [w556]
          tunnel: w508 -> [w555]
          tunnel: w510 -> [w567]
          tunnel: [w569] -> w528
          tunnel: w509 -> [w568]
          tunnel: [w570] -> w527
          tunnel: w528 -> [w582]
          tunnel: [w583] -> w526
          tunnel: w527 -> [w581]
          tunnel: [w584] -> w525
          tunnel: w526 -> [w589]
          tunnel: [w588] -> w524
          tunnel: w525 -> [w590]
          tunnel: [w591] -> w523
          tunnel: w524 -> [w602]
          tunnel: [w601] -> w522
          tunnel: w523 -> [w603]
          tunnel: [w604] -> w521
          tunnel: w522 -> [w621]
          tunnel: [w620] -> w520
          tunnel: w521 -> [w622]
          tunnel: [w623] -> w519
          tunnel: w520 -> [w639]
          tunnel: [w641] -> w518
          tunnel: w519 -> [w640]
          tunnel: [w642] -> w517
          tunnel: w518 -> [w654]
          tunnel: [w652] -> w506
          tunnel: w517 -> [w655]
          tunnel: [w653] -> w504
          tunnel: w506 -> [w668]
          tunnel: [w667] -> w505
          tunnel: w504 -> [w670]
          tunnel: [w669] -> w503
          tunnel: w505 -> [w691]
          tunnel: w503 -> [w692]
          tunnel: [w677] -> w514
          tunnel: [w681] -> w513
          tunnel: w514 -> [w707]
          tunnel: w513 -> [w706]
          tunnel: [w705] -> w512
          tunnel: [w704] -> w511
          tunnel: [w723] -> w530
          tunnel: [w722] -> w529
          tunnel: w512 -> [w717]
          tunnel: w511 -> [w716]
          tunnel: w530 -> [w793]
          tunnel: w529 -> [w792]
          tunnel: [w789] -> w516
          tunnel: [w788] -> w515
          tunnel: w516 -> [w821]
          tunnel: w515 -> [w820]
          frame #0 {
            n227 = Open/Create/Replace File(operation (0:open)=4) -> (refnum out=w541:refnum<file>, error out=w540:errorcluster)  [unwired: 5 in, 1 out]
            n228 = Get Date/Time In Seconds() -> (seconds since 1Jan1904=w535:timestamp)
            n229 = Format Into String(format string="%s,%s,%s,%<%d/%m/%Y>T,%s,%s\\n", initial string=w541, error in=w540, "Experiment Type", "Experiment Name", "Date:" ("Command"), w535, "Operator:" ("Command"), "Operator Name") -> (resulting string=w532:refnum<file>, error out=w531:errorcluster)
          }
          frame #1 {
            n230 = Format Into String(format string="%s,%s,%s,%s,%s,,,,%s,%s\\n%s,%s,,,", initial string=w556, error in=w555, "Sugar Source" ("Command"), "Additive Type" ("Command"), "Seeding Method" ("Command"), "Seed Type" ("Command"), "Time Interval (MM:SS)" ("Command"), "Temp. Julabo Steel [°C]" ("Command"), "Temp. Julabo Glass [°C]" ("Command"), "Sugar Source", "Additives") -> (resulting string=w544:refnum<file>, error out=w543:errorcluster)
          }
          frame #2 {
            n231 = property on="Time Interval" class="DigNum (strict)"() -> ("Value"=w565:dbl)  [unwired: 2 in, 2 out]
            n232 = Format Into String(format string="%<%M:%S>t,,,,\\n%s,,,%s,,,\\n%s,%s,%s,%s,%s,%s\\n", initial string=w568, error in=w567, w565, "Syrup Parameters" ("Command"), "Crystallization Parameters" ("Command"), "Parameter" ("Command"), "Unit" ("Command"), "Value" ("Command"), "Parameter" ("Command"), "Unit" ("Command"), "Value" ("Command")) -> (resulting string=w570:refnum<file>, error out=w569:errorcluster)
          }
          frame #3 {
            n233 = property on="Total Amount Added [gr]" class="DigNum (strict)"() -> ("Value"=w571:dbl)  [unwired: 2 in, 2 out]
            n234 = Format Into String(format string="%s,%s,,%s,%s,,\\n%s,%s,,%s,%s,%.1f\\n", initial string=w581, error in=w582, "Total Syrup" ("Command"), "g" ("Command"), "Total Weight" ("Command"), "g" ("Command"), "Additive Amount" ("Command"), "g" ("Command"), "Starting Weight" ("Command"), "g" ("Command"), w571) -> (resulting string=w584:refnum<file>, error out=w583:errorcluster)
          }
          frame #4 {
            n235 = Format Into String(format string="%s,%s,%.2f,%s,%s,,\\n%s,%s,%.1f,%s,%s,,\\n", initial string=w590, error in=w589, "%Additive" ("Command"), "%" ("Command"), "Percentage [%]", "Feeding Weight" ("Command"), "g" ("Command"), "Syrup °Bx by Manual RF" ("Command"), "Brix" ("Command"), "Syrup °Bx by Manual RF", "Weight Ratio" ("Command"), "%" ("Command")) -> (resulting string=w591:refnum<file>, error out=w588:errorcluster)
          }
          frame #5 {
            n236 = Format Into String(format string="%s,%s,,%s,%s,,\\n%s,%s,%.1f,%s,%s,,\\n", initial string=w603, error in=w602, "Purity" ("Command"), "%" ("Command"), "Agitator" ("Command"), "RPM" ("Command"), "Syrup + Additive °Bx by Manual RF" ("Command"), "Brix" ("Command"), "°Bx DM", "Seed Size" ("Command"), "um" ("Command")) -> (resulting string=w604:refnum<file>, error out=w601:errorcluster)
          }
          frame #6 {
            n237 = property on="°Bx In-Line" class="DigNum (strict)"() -> ("Value"=w619:dbl)  [unwired: 2 in, 2 out]
            n238 = Format Into String(format string="%s,%s,%.2f,%s,%s,,\\n%s,%s,%<%H:%M>t,%s,%s,,\\n", initial string=w622, error in=w621, "°BX by In-Line RF" ("Command"), "Brix" ("Command"), w619, "Seeding Temp." ("Command"), "°C" ("Command"), "Mixing Time" ("Command"), "HH:MM" ("Command"), "Mixing Time", "Seeding °BX" ("Command"), "Brix" ("Command")) -> (resulting string=w623:refnum<file>, error out=w620:errorcluster)
          }
          frame #7 {
            n239 = Format Into String(format string="%s,%s,%d,%s,%s,,\\n%s,%s,%.1f,%s,%s,,\\n", initial string=w640, error in=w639, "Mixing Speed" ("Command"), "RPM" ("Command"), "Mixing RPM", "Seeding Amount" ("Command"), "g" ("Command"), "Temp." ("Command"), "°C" ("Command"), "Temp. [°C]", "Seeding Supersaturation" ("Command"), "NA" ("Command")) -> (resulting string=w642:refnum<file>, error out=w641:errorcluster)
          }
          frame #8 {
            n240 = Format Into String(format string="%s,%s,%.2f,%s,%s,,\\n,,,%s,%s,%<%M:%S>t\\n", initial string=w655, error in=w654, "pH" ("Command"), "NA" ("Command"), "pH", "Seeding Time" ("Command"), "HH:MM:SS" ("Command"), "Silverson Duration" ("Command"), "MM:SS" ("Command"), "Silverson Duration (MM:SS)") -> (resulting string=w653:refnum<file>, error out=w652:errorcluster)
          }
          frame #9 {
            n241 = Format Into String(format string=",,,%s,%s,%d\\n,,,%s,%s,%<%H:%M>T\\n\\n\\n%s,,,,,,,%s,,,,,,,,,,,,,%s\\n", initial string=w670, error in=w668, "Silverson Speed" ("Command"), "RPM" ("Command"), "Speed RPM", "Loading Delay" ("Command"), "HH:MM" ("Command"), "Loading Delay", "Material Data" ("Command"), "Equipment" ("Command"), "Comments" ("Command")) -> (resulting string=w669:refnum<file>, error out=w667:errorcluster)
          }
          frame #10 {
            n242 = Format Into String(format string="%s,%s,%s,%s,%s,%s,%s,%s,%s,%s,,%s,%s,%s,%s,,%s,,%s,%s\\n", initial string=w692, error in=w691, "Time (HH:MM:SS)" ("Command"), "Recording Time [sec]" ("Command"), "Syrup Feed" ("Command"), "Mass Flow" ("Command"), "Water Evaporation" ("Command"), "Evaporation Rate" ("Command"), "Total Mass" ("Command"), "Vacuum" ("Command"), "PT-100" ("Command"), "Refractometer" ("Command"), "Torque" ("Command"), "Pump" ("Command"), "TS Calculated" ("Command"), "Brix Change" ("Command"), "Supersaturation" ("Command"), "Julabo Stainless Steel" ("Command"), "Julabo Glass" ("Command")) -> (resulting string=w677:refnum<file>, error out=w681:errorcluster)
          }
          frame #11 {
            n243 = Format Into String(format string=",,%s,%s,%s,%s,%s,%s,%s,%s,%s,%s,%s,%s,%s,%s,%s,%s,%s,%s\\n", initial string=w707, error in=w706, "g" ("Command"), "g/Min" ("Command"), "g" ("Command"), "g/Min" ("Command"), "g" ("Command"), "mbar" ("Command"), "Temp. [°C]" ("Command"), "% Brix" ("Command"), "Temp. [°C]" ("Command"), "Ncm" ("Command"), "RPM" ("Command"), "% TS" ("Command"), "% Brix" ("Command"), "% Brix_r" ("Command"), "Ref" ("Command"), "TS" ("Command"), "Temp [°C]" ("Command"), "Temp [°C]" ("Command")) -> (resulting string=w705:refnum<file>, error out=w704:errorcluster)
          }
          frame #12 {
            n244 = while {
              shift-right: [w733] -> w723
              shift-left: w717 -> [w734]
              tunnel: w716 -> [w732]
              tunnel: [w731] -> w722
              shift-right: ["Time Interval"] -> _
              shift-left: 0.0 ("Time Interval") -> [w724]
              shift-right: [w728] -> w719
              shift-left: errorcluster {"status"=FALSE, "code"=0, "source"=""} ("error out") -> [w737]
              shift-right: [w725] -> _
              shift-left: 0.0 -> [w726]
              stop <- w727 stop-if-true
              n245 = call "Elapsed Time2"("Time Target (s)"=w724, "Auto Reset"=TRUE, "error in (no error)"=w737) -> ("Time has Elapsed"=w738:bool, "error out"=w736:errorcluster)  [unwired: 9 in, 6 out]
              n246 = case shown="True" w738 {
                tunnel: [w746 w755] -> w728
                tunnel: w736 -> [w746 w755]
                tunnel: w734 -> [w745 w759]
                tunnel: [w745 w758] -> w733
                tunnel: w732 -> [w744 w757]
                tunnel: [w744 w756] -> w731
                tunnel: w726 -> [w743 w752]
                tunnel: [w743 w753] -> w725
                tunnel: w724 -> [_ w750]
                frame False {
                }
                frame True {
                  n247 = Multiply(x=w752, y=w750) -> (x*y=w751:dbl)
                  n248 = Add(x=1.0, y=w752) -> (x+y=w753:dbl)
                  n249 = property on="Condensate Weight [gr]" class="Slide (strict)"() -> ("Value"=w761:dbl)  [unwired: 2 in, 2 out]
                  n250 = property on="Process" class="DigNum (strict)"() -> ("Value"=w762:dbl)  [unwired: 2 in, 2 out]
                  n251 = property on="Tank's Solution\nWeight [gr]" class="Slide (strict)"() -> ("Value"=w763:dbl)  [unwired: 2 in, 2 out]
                  n252 = property on="°Bx" class="DigNum (strict)"() -> ("Value"=w765:dbl)  [unwired: 2 in, 2 out]
                  n253 = property on="Speed RPM" class="DigNum (strict)"() -> ("Value"=w747:dbl)  [unwired: 2 in, 2 out]
                  n254 = property on="Internal Temp." class="Slide (strict)"() -> ("Value"=w748:dbl)  [unwired: 2 in, 2 out]
                  n255 = property on="Internal Temp." class="Slide (strict)"() -> ("Value"=w749:dbl)  [unwired: 2 in, 2 out]
                  n256 = property on="Temp. [°C]" class="DigNum (strict)"() -> ("Value"=w766:dbl)  [unwired: 2 in, 2 out]
                  n257 = property on="Torque [Ncm]" class="Str"() -> ("Value"=w767:string)  [unwired: 2 in, 2 out]
                  n258 = property on="Current\nPressure\n[mbar]" class="Knob (strict)"() -> ("Value"=w764:dbl)  [unwired: 2 in, 2 out]
                  n259 = Get Date/Time In Seconds() -> (seconds since 1Jan1904=w769:timestamp)
                  n260 = property on="Temp. [°C]" class="DigNum (strict)"() -> ("Value"=w768:dbl)  [unwired: 2 in, 2 out]
                  n261 = Format Into String(format string="%<%H:%M:%S>T,%d,,,%.1f,%.3f,%.1f,%.1f,%.1f,%.2f,%.1f,%s,%d,%.1f,%.1f\\n", initial string=w759, error in=w757, w769, w751, w761, w762, w763, w764, w768, w765, w766, w767, w747, w748, w749) -> (resulting string=w758:refnum<file>, error out=w756:errorcluster)
                }
              }
              n262 = property on="Stop Program" class="Bool (strict)"() -> ("Value"=w742:bool)  [unwired: 2 in, 2 out]
              n263 = property on="Start/Stop\nRecording" class="Bool (strict)"() -> ("Value"=w740:bool)  [unwired: 2 in, 2 out]
              n264 = Wait (ms)(milliseconds to wait=u32 10) -> ()  [unwired: 1 out]
              n265 = Not(x=w740) -> (.not. x?=w741:bool)
              n266 = Or(x=w742, y=w741) -> (x .or. y?=w729:bool)
              n267 = Or(x=w728, y=w729) -> (x .or. y?=w727:bool)
            }
            n268 = call <vilib>:"Simple Error Handler.vi"("error in (no error)"=w719) -> ()  [unwired: 4 in, 5 out]
          }
          frame #13 {
            n269 = Format Into String(format string="\\n%s,%s,%s,%s,%s,%s,%s,%s,%s\\n", initial string=w793, error in=w792, "Centrifugation Duration [MM:SS]" ("Command"), "Centrifugation Speed" ("Command"), "Loading 1st Cycle [gr]" ("Command"), "Loading 2nd Cycle [gr]" ("Command"), "Feed 1st Cycle [gr]" ("Command"), "Feed 2nd Cycle [gr]" ("Command"), "Emptying 1st Cycle [gr]" ("Command"), "Emptying 2nd Cycle [gr]" ("Command"), "Yield [%]" ("Command")) -> (resulting string=w795:refnum<file>, error out=w794:errorcluster)
            n270 = Format Into String(format string="%<%M:%S>t,%d,%.2f,%.2f,%.2f,%.2f,%.2f,%.2f,%.2f\\n\\n", initial string=w795, error in=w794, "Cent. Duration (MM:SS)", "Speed", "Loading 1st\nCycle [gr]", "Loading 2nd\nCycle [gr]", "Feed 1st Cycle [gr]", "Feed 2nd Cycle [gr]", "Emptying 1st\nCycle [gr]", "Emptying 2nd\nCycle [gr]", "Yield [%]") -> (resulting string=w789:refnum<file>, error out=w788:errorcluster)
          }
          frame #14 {
            n271 = property on="Seeding Julabo SS Temp. [°C]" class="DigNum (strict)"() -> ("Value"=w804:dbl)  [unwired: 2 in, 2 out]
            n272 = property on="Seeding Julabo Glass Temp. [°C]" class="DigNum (strict)"() -> ("Value"=w803:dbl)  [unwired: 2 in, 2 out]
            n273 = property on="Amount of Sugar [gr]" class="DigNum (strict)"() -> ("Value"=w812:dbl)  [unwired: 2 in, 2 out]
            n274 = property on="Amount of Dry Substance\n[gr]" class="DigNum (strict)"() -> ("Value"=w813:dbl)  [unwired: 2 in, 2 out]
            n275 = property on="Seeding RPM" class="DigNum (strict)"() -> ("Value"=w811:dbl)  [unwired: 2 in, 2 out]
            n276 = property on="Total Amount Added [gr]" class="DigNum (strict)"() -> ("Value"=w814:dbl)  [unwired: 2 in, 2 out]
            n277 = Divide(x=w812, y=w813) -> (x/y=w802:dbl)
            n278 = Multiply(x=w802, y=100.0) -> (x*y=w801:dbl)
            n279 = Format Into String(format string="%s,%.1f,%.1f,%.1f,%.2f,%d,%s,", initial string=w821, error in=w820, "$@!" ("Command"), w804, w803, w814, w801, w811, "Size (um)") -> (resulting string=w819:refnum<file>, error out=w818:errorcluster)
            n280 = property on="Seeding Temp. [°C]" class="DigNum (strict)"() -> ("Value"=w810:dbl)  [unwired: 2 in, 2 out]
            n281 = property on="Seeding °Bx" class="DigNum (strict)"() -> ("Value"=w809:dbl)  [unwired: 2 in, 2 out]
            n282 = property on="Amount [gr]" class="DigNum (strict)"() -> ("Value"=w808:dbl)  [unwired: 2 in, 2 out]
            n283 = property on="Seeding Kss" class="DigNum (strict)"() -> ("Value"=w807:dbl)  [unwired: 2 in, 2 out]
            n284 = property on="Seed Time" class="AbsTime (strict)"() -> ("Value"=w806:timestamp)  [unwired: 2 in, 2 out]
            n285 = property on="Syrup Added [gr]" class="Slide (strict)"() -> ("Value"=w799:dbl)  [unwired: 2 in, 2 out]
            n286 = Format Into String(format string="%.1f,%.2f,%.1f,%.2f,%<%H:%M:%S>T,%.1f,%s,%s\\n", initial string=w819, error in=w818, w810, w809, w808, w807, w806, w799, "Method", "Seed Type") -> (resulting string=w817:refnum<file>)  [unwired: 1 out]
            n287 = Close File(refnum=w817) -> ()  [unwired: 1 in, 2 out]
          }
        }
      }
    }
  }
  n288 = while {
    stop <- w823 stop-if-true
    n289 = property on="Stop Program" class="Bool (strict)"() -> ("Value"=w823:bool)  [unwired: 2 in, 2 out]
    n290 = Wait (ms)(milliseconds to wait=u32 1000) -> ()  [unwired: 1 out]
    n291 = case shown="True" "Condensate Balance" {
      frame False {
      }
      frame True {
        n292 = flat-sequence {
          tunnel: [w853] -> w830
          tunnel: [w854] -> w829
          tunnel: [w843] -> w828
          tunnel: w830 -> [w862]
          tunnel: w829 -> [w861]
          tunnel: w828 -> [w858]
          tunnel: [w864] -> w827
          tunnel: [w863] -> w826
          tunnel: [w858] -> w825
          tunnel: w827 -> [w973]
          tunnel: w826 -> [w972]
          tunnel: w825 -> [w975]
          frame #0 {
            w839 = u16 10 items=["1.0"=10, "1.5"=15, "2.0"=20] ("stop bits (10: 1 bit)")
            n293 = control-ref of="Boolean 17"() -> (w852:refnum<vi>)
            n294 = control-ref of="Boolean 16"() -> (w851:refnum<vi>)
            n295 = control-ref of="Boolean 15"() -> (w850:refnum<vi>)
            n296 = control-ref of="Boolean 14"() -> (w849:refnum<vi>)
            n297 = control-ref of="Boolean 13"() -> (w848:refnum<vi>)
            n298 = control-ref of="Boolean 12"() -> (w847:refnum<vi>)
            n299 = control-ref of="Boolean 11"() -> (w846:refnum<vi>)
            n300 = control-ref of="Boolean 10"() -> (w845:refnum<vi>)
            n301 = Build Array(w852, w851, w850, w849, w848, w847, w846, w845) -> (w844:refnum<vi>[])
            n302 = for {
              tunnel: w844 -> [w857] mode=indexing
              tunnel: [w855] -> w843 mode=indexing
              n303 = property class="Bool (strict)"(reference=w857, "Value"=FALSE) -> (reference out=w855:refnum<vi>)  [unwired: 1 in, 1 out]
            }
            n304 = call-poly "VISA Configure Serial Port"("VISA resource name"="Condensate Balance", "baud rate (9600)"=u32 9600, "data bits (8)"=u16 8, "parity (0:none)"=enum16{"None", "Odd", "Even", "Mark", "Space"}."None", "stop bits (10: 1 bit)"=w839, "flow control (0:none)"=enum16{"None", "XON/XOFF", "RTS/CTS", "DTR/DSR"}."None" ("parity (0:none)")) -> ("VISA resource name out"=w854:refnum<visa-resource-name>, "error out"=w853:errorcluster)  [unwired: 8 in]
            n305 = property on="5 min." class="DigNum (strict)"("Value"=nan ("5 min. acc.")) -> ()  [unwired: 2 in, 2 out]
            n306 = property on="20 min." class="DigNum (strict)"("Value"=nan ("5 min. acc.")) -> ()  [unwired: 2 in, 2 out]
            n307 = property on="Process" class="DigNum (strict)"("Value"=nan ("5 min. acc.")) -> ()  [unwired: 2 in, 2 out]
            n308 = property on="1 min. TS" class="DigNum (strict)"("Value"=nan ("1 min. TS")) -> ()  [unwired: 2 in, 2 out]
            n309 = property on="Theoretical 5 min. TS" class="DigNum (strict)"("Value"=nan ("1 min. TS")) -> ()  [unwired: 2 in, 2 out]
            n310 = property on="Condensate Balance Restart" class="Bool (strict)"("Value"=FALSE ("Condensate Balance Restart")) -> ()  [unwired: 2 in, 2 out]
          }
          frame #1 {
            n311 = while {
              tunnel: [w867] -> w864
              tunnel: [w866] -> w863
              tunnel: w862 -> [w894]
              tunnel: w861 -> [w895]
              shift-right: [w890] -> _
              shift-left: dbl[] [] -> [w888]
              shift-right: [w880] -> _
              shift-left: dbl[] [] -> [w879]
              tunnel: w858 -> [w877]
              i -> [w881]
              stop <- w903 stop-if-true
              n312 = property on="5 min." class="DigNum (strict)"() -> ("Value"=w874:dbl)  [unwired: 2 in, 2 out]
              n313 = Not A Number/Path/Refnum?(number/path/refnum=w874) -> (NaN/Path/Refnum?=w875:bool)
              n314 = Concatenate Strings("Q" ("Command"), "\r", "\n") -> (w899:string)
              n315 = Wait (ms)(milliseconds to wait=u32 200) -> ()  [unwired: 1 out]
              n316 = case shown="True" w875 {
                tunnel: w877 -> [_ w909]
                tunnel: w874 -> [_ w907]
                frame False {
                }
                frame True {
                  n317 = Greater?(x=w907, y=2.0) -> (0:w910:bool)
                  n318 = case shown="True" w910 {
                    tunnel: w909 -> [w911 w915]
                    frame False {
                      n319 = for {
                        tunnel: w911 -> [w914] mode=indexing
                        tunnel: [w912] -> _ mode=indexing
                        n320 = property class="Bool (strict)"(reference=w914, "Value"=FALSE) -> (reference out=w912:refnum<vi>)  [unwired: 1 in, 1 out]
                      }
                    }
                    frame True {
                      n321 = for {
                        tunnel: w915 -> [w918] mode=indexing
                        tunnel: [w916] -> _ mode=indexing
                        n322 = property class="Bool (strict)"(reference=w918, "Value"=TRUE) -> (reference out=w916:refnum<vi>)  [unwired: 1 in, 1 out]
                      }
                    }
                  }
                }
              }
              n323 = VISA Write(VISA resource name=w895, write buffer=w899, error in (no error)=w894) -> (VISA resource name out=w901:refnum<visa-resource-name>, error out=w900:errorcluster)  [unwired: 1 out]
              n324 = property on="Condensate Balance" class="Bool (strict)"() -> ("Value"=w902:bool)  [unwired: 2 in, 2 out]
              n325 = flat-sequence {
                tunnel: w901 -> [w971]
                tunnel: w900 -> [w970]
                tunnel: [w971] -> w869
                tunnel: [w970] -> w868
                frame #0 {
                  n326 = Wait (ms)(milliseconds to wait=u32 100) -> ()  [unwired: 1 out]
                }
              }
              n327 = Not(x=w902) -> (.not. x?=w889:bool)
              n328 = property on="Stop Program" class="Bool (strict)"() -> ("Value"=w904:bool)  [unwired: 2 in, 2 out]
              n329 = Or(x=w889, y=w904) -> (x .or. y?=w903:bool)
              n330 = VISA Read(VISA resource name=w869, byte count=u32 30, error in (no error)=w868) -> (VISA resource name out=w872:refnum<visa-resource-name>, read buffer=w870:string, error out=w871:errorcluster)  [unwired: 1 out]
              n331 = call <instrlib>:"A&D Data Separate.vi"("error in (no error)"=w871, "Received Data"=w870, "VISA resource name"=w872) -> ("error out"=w866:errorcluster, "Value"=w865:dbl, "VISA resource name out"=w867:refnum<visa-resource-name>)  [unwired: 4 in, 2 out]
              "Condensate Weight [gr]" <- w865
              n332 = case shown="True" "Seeds Added" {
                tunnel: w888 -> [_ w932]
                tunnel: w881 -> [_ w931]
                frame False {
                }
                frame True {
                  n333 = property on="Process" class="DigNum (strict)"() -> ("Value"=w933:dbl)  [unwired: 2 in, 2 out]
                  n334 = Not A Number/Path/Refnum?(number/path/refnum=w933) -> (NaN/Path/Refnum?=w934:bool)
                  n335 = case shown="False" w934 {
                    tunnel: w932 -> [w946 _]
                    tunnel: w931 -> [w937 w947]
                    frame False {
                      n336 = Subtract(x=w937, y=1) -> (x-y=w938:i32)
                      n337 = property on="Process Start" class="DigNum (strict)"() -> ("Value"=w936:i32)  [unwired: 2 in, 2 out]
                      n338 = Index Array(array=w946, index #1=w936, index #2=w938) -> (element #1=w941:dbl, element #2=w940:dbl)
                      n339 = Subtract(x=w937, y=w936) -> (x-y=w944:i32)
                      n340 = Subtract(x=w940, y=w941) -> (x-y=w945:dbl)
                      n341 = Divide(x=w944, y=300) -> (x/y=w942:dbl)
                      n342 = Divide(x=w945, y=w942) -> (x/y=→"Process" →"Process 2":dbl)
                    }
                    frame True {
                      n343 = property on="Process" class="DigNum (strict)"("Value"=0.0 ("Process avg.")) -> ()  [unwired: 2 in, 2 out]
                      "Process Start" <- w947
                    }
                  }
                }
              }
              n344 = Build Array(w865) -> (w876:dbl[])
              n345 = Add(x=w881, y=1) -> (x+y=w884:i32)
              n346 = Insert Into Array(array=w888, index=w881, new element=w876) -> (w890:dbl[])
              n347 = Greater?(x=w884, y=299) -> (0:w883:bool)
              n348 = Add(x=w881, y=1) -> (x+y=w891:i32)
              n349 = Greater?(x=w891, y=1499) -> (0:w892:bool)
              n350 = property on="Dry Substance [%]" class="Slide (strict)"() -> ("Value"=w882:dbl)  [unwired: 2 in, 2 out]
              n351 = case shown="True" w892 {
                tunnel: w890 -> [_ w952]
                tunnel: w881 -> [_ w953]
                frame False {
                }
                frame True {
                  n352 = Greater?(x=w953, y=5999) -> (0:w954:bool)
                  n353 = Subtract(x=w953, y=1499) -> (x-y=w959:i32)
                  n354 = case shown="True" w954 {
                    tunnel: w953 -> [_ w962]
                    tunnel: w952 -> [_ w961]
                    frame False {
                    }
                    frame True {
                      n355 = Subtract(x=w962, y=5999) -> (x-y=w968:i32)
                      n356 = Index Array(array=w961, index #1=w962, index #2=w968) -> (element #1=w965:dbl, element #2=w966:dbl)
                      n357 = Subtract(x=w965, y=w966) -> (x-y=w964:dbl)
                      n358 = Divide(x=w964, y=20.0) -> (x/y=→"20 min.":dbl)
                    }
                  }
                  n359 = Index Array(array=w952, index #1=w953, index #2=w959) -> (element #1=w956:dbl, element #2=w957:dbl)
                  n360 = Subtract(x=w956, y=w957) -> (x-y=w951:dbl)
                  n361 = Divide(x=w951, y=5.0) -> (x/y=→"5 min.":dbl)
                }
              }
              n362 = Build Array(w882) -> (w887:dbl[])
              n363 = Insert Into Array(array=w879, index=w881, new element=w887) -> (w880:dbl[])
              n364 = case shown="True" w883 {
                tunnel: w880 -> [_ w920]
                tunnel: w881 -> [_ w919]
                frame False {
                }
                frame True {
                  n365 = flat-sequence {
                    tunnel: w920 -> [w923]
                    tunnel: w919 -> [w922]
                    frame #0 {
                      n366 = Subtract(x=w922, y=299) -> (x-y=w927:i32)
                      n367 = Index Array(array=w923, index #1=w922, index #2=w927) -> (element #1=w924:dbl, element #2=w925:dbl)
                      n368 = Subtract(x=w924, y=w925) -> (x-y=→"1 min. TS":dbl)
                    }
                    frame #1 {
                      n369 = property on="1 min. TS" class="DigNum (strict)"() -> ("Value"=w930:dbl)  [unwired: 2 in, 2 out]
                      n370 = Multiply(x=w930, y=5.0) -> (x*y=→"Theoretical 5 min. TS":dbl)
                    }
                  }
                }
              }
            }
          }
          frame #2 {
            n371 = for {
              tunnel: w975 -> [w977] mode=indexing
              n372 = property class="Bool (strict)"(reference=w977, "Value"=FALSE) -> ()  [unwired: 1 in, 2 out]
            }
            n373 = VISA Close(VISA resource name=w973, error in (no error)=w972) -> (error out=w974:errorcluster)
            n374 = call <vilib>:"Simple Error Handler.vi"("error in (no error)"=w974) -> ()  [unwired: 1 in, 8 out]
          }
          frame #3 {
            "Condensate Balance Restart" <- TRUE ("Condensate Balance Restart")
          }
        }
      }
    }
  }
  n375 = while {
    stop <- w980 stop-if-true
    n376 = property on="Stop Program" class="Bool (strict)"() -> ("Value"=w980:bool)  [unwired: 2 in, 2 out]
    n377 = Wait (ms)(milliseconds to wait=u32 1000) -> ()  [unwired: 1 out]
    n378 = case shown="True" "Peristaltic Balance" {
      frame False {
      }
      frame True {
        n379 = flat-sequence {
          tunnel: [w1000] -> w985
          tunnel: [w1001] -> w984
          tunnel: w985 -> [w1005]
          tunnel: w984 -> [w1004]
          tunnel: [w1007] -> w983
          tunnel: [w1006] -> w982
          tunnel: w983 -> [w1096]
          tunnel: w982 -> [w1095]
          frame #0 {
            w996 = u16 10 items=["1.0"=10, "1.5"=15, "2.0"=20] ("stop bits (10: 1 bit)")
            n380 = property on="Dry Substance [%]" class="DigNum (strict)"("Value"=0.0 ("Dry Substance [%]"), "NumText.BGColor"=u32 16711680 ("Numeric Text.Text Colors:BG Color")) -> ()  [unwired: 2 in, 2 out]
            n381 = property on="Purity (0.92-1.0)" class="DigNum (strict)"("Value"=0.0 ("Purity (0.92-1.0)"), "NumText.BGColor"=u32 16711680 ("Numeric Text.Text Colors:BG Color")) -> ()  [unwired: 2 in, 2 out]
            n382 = call-poly "VISA Configure Serial Port"("VISA resource name"="Peristaltic Balance", "baud rate (9600)"=u32 9600, "data bits (8)"=u16 8, "parity (0:none)"=enum16{"None", "Odd", "Even", "Mark", "Space"}."None", "stop bits (10: 1 bit)"=w996, "flow control (0:none)"=enum16{"None", "XON/XOFF", "RTS/CTS", "DTR/DSR"}."None" ("parity (0:none)")) -> ("VISA resource name out"=w1001:refnum<visa-resource-name>, "error out"=w1000:errorcluster)  [unwired: 8 in]
            n383 = property on="Addition Rate 1 min. [gr/min]" class="DigNum (strict)"("Value"=0.0 ("Addition Rate 1 min. [gr/min]")) -> ()  [unwired: 2 in, 2 out]
            n384 = property on="Syrup Added [gr]" class="Slide (strict)"("Value"=0.0 ("Syrup Added [gr]")) -> ()  [unwired: 2 in, 2 out]
            n385 = property on="Peristaltic Balance Restart" class="Bool (strict)"("Value"=FALSE ("Peristaltic Balance Restart")) -> ()  [unwired: 2 in, 2 out]
            n386 = property on="Theoretical Addition Rate [gr/min]" class="DigNum (strict)"("Value"=nan ("5 min. acc.")) -> ()  [unwired: 2 in, 2 out]
          }
          frame #1 {
            n387 = while {
              tunnel: [w1013] -> w1007
              tunnel: [w1012] -> w1006
              tunnel: w1005 -> [w1054]
              tunnel: w1004 -> [w1055]
              shift-right: [w1048] -> _
              shift-left: dbl[] [] -> [w1049]
              shift-right: [w1008] -> _
              shift-left: 0.0 -> [w1009]
              i -> [w1047]
              stop <- w1057 stop-if-true
              n388 = property on="Purity (0.92-1.0)" class="DigNum (strict)"() -> ("Value"=w1034:dbl)  [unwired: 2 in, 2 out]
              n389 = property on="Dry Substance [%]" class="DigNum (strict)"() -> ("Value"=w1031:dbl)  [unwired: 2 in, 2 out]
              n390 = Not Equal?(x=w1034, y=0.0) -> (x != y?=w1033:bool)
              n391 = Not Equal?(x=0.0 ("y"), y=w1031) -> (x != y?=w1026:bool)
              n392 = property on="5 min." class="DigNum (strict)"() -> ("Value"=w1036:dbl)  [unwired: 2 in, 2 out]
              n393 = Divide(x=w1031, y=100.0) -> (x/y=w1027:dbl)
              n394 = case shown="True" w1033 {
                frame False {
                }
                frame True {
                  n395 = property on="Purity (0.92-1.0)" class="DigNum (strict)"("NumText.BGColor"=u32 65280 ("Numeric Text.Text Colors:BG Color")) -> ()  [unwired: 2 in, 2 out]
                }
              }
              n396 = case shown="True" w1026 {
                frame False {
                }
                frame True {
                  n397 = property on="Dry Substance [%]" class="DigNum (strict)"("NumText.BGColor"=u32 65280 ("Numeric Text.Text Colors:BG Color")) -> ()  [unwired: 2 in, 2 out]
                }
              }
              n398 = Not A Number/Path/Refnum?(number/path/refnum=w1036) -> (NaN/Path/Refnum?=w1039:bool)
              n399 = Concatenate Strings("SI" ("Command"), "\r", "\n") -> (w1023:string)
              n400 = Subtract(x=1.0, y=w1027) -> (x-y=w1028:dbl)
              n401 = Not(x=w1039) -> (.not. x?=w1038:bool)
              n402 = VISA Write(VISA resource name=w1055, write buffer=w1023, error in (no error)=w1054) -> (VISA resource name out=w1025:refnum<visa-resource-name>, error out=w1024:errorcluster)  [unwired: 1 out]
              n403 = And(x=w1026, y=w1038) -> (x .and. y?=w1037:bool)
              n404 = flat-sequence {
                tunnel: w1025 -> [w1081]
                tunnel: w1024 -> [w1080]
                tunnel: [w1081] -> w1010
                tunnel: [w1080] -> w1011
                frame #0 {
                  n405 = Wait (ms)(milliseconds to wait=u32 100) -> ()  [unwired: 1 out]
                }
              }
              n406 = case shown="True" w1037 {
                tunnel: w1028 -> [_ w1085]
                tunnel: w1036 -> [_ w1084]
                frame False {
                  n407 = property on="Theoretical Addition Rate [gr/min]" class="DigNum (strict)"("Value"=nan ("5 min. acc.")) -> ()  [unwired: 2 in, 2 out]
                }
                frame True {
                  n408 = Divide(x=w1084, y=w1085) -> (x/y=→"Theoretical Addition Rate [gr/min]":dbl)
                }
              }
              n409 = property class="Instr"(reference=w1010, error in=w1011) -> (reference out=w1017:refnum<visa-resource-name>, error out=w1018:errorcluster, "Serial Settings:Number of Bytes at Serial Port"=w1015:u32)
              n410 = Greater Or Equal?(x=w1015, y=u32 17) -> (x >= y?=w1016:bool)
              n411 = case shown="False" w1016 {
                tunnel: w1015 -> [_ w1076]
                tunnel: w1018 -> [w1061 w1075]
                tunnel: w1017 -> [w1062 w1074]
                tunnel: [w1062 w1070] -> w1013
                tunnel: [w1061 w1069] -> w1012
                tunnel: [w1060 w1064] -> w1008
                tunnel: w1009 -> [w1060 w1063]
                frame False {
                }
                frame True {
                  n412 = VISA Read(VISA resource name=w1074, byte count=w1076, error in (no error)=w1075) -> (VISA resource name out=w1070:refnum<visa-resource-name>, read buffer=w1073:string, error out=w1069:errorcluster)  [unwired: 1 out]
                  n413 = String Subset(string=w1073, offset (0)=9) -> (substring=w1072:string)  [unwired: 1 in]
                  n414 = Fract/Exp String To Number(string=w1072) -> (offset past number=w1068:i32, number=w1065:dbl)  [unwired: 3 in]
                  n415 = Less?(x=0, y=w1068) -> (x < y?=w1066:bool)
                  n416 = case shown="False" w1066 {
                    tunnel: [w1077 w1078] -> w1064
                    tunnel: w1065 -> [_ w1078]
                    tunnel: w1063 -> [w1077 _]
                    frame False {
                    }
                    frame True {
                    }
                  }
                }
              }
              n417 = Add(x=w1047, y=1) -> (x+y=w1044:i32)
              n418 = Quotient & Remainder(x=w1044, y=300) -> (x-y*floor(x/y)=w1042:i32)  [unwired: 1 out]
              n419 = Greater?(x=w1044, y=299) -> (0:w1045:bool)
              n420 = Equal?(x=0, y=w1042) -> (x = y?=w1040:bool)
              n421 = And(x=w1045, y=w1040) -> (x .and. y?=w1046:bool)
              n422 = property on="Peristaltic Balance" class="Bool (strict)"() -> ("Value"=w1056:bool)  [unwired: 2 in, 2 out]
              n423 = Wait (ms)(milliseconds to wait=u32 200) -> ()  [unwired: 1 out]
              n424 = property on="Stop Program" class="Bool (strict)"() -> ("Value"=w1058:bool)  [unwired: 2 in, 2 out]
              n425 = Not(x=w1056) -> (.not. x?=w1053:bool)
              n426 = Or(x=w1053, y=w1058) -> (x .or. y?=w1057:bool)
              n427 = Build Array(w1008) -> (w1052:dbl[])
              n428 = Absolute Value(x=w1008) -> (abs(x)=→"Syrup Added [gr]":dbl)
              n429 = Insert Into Array(array=w1049, index=w1047, new element=w1052) -> (w1048:dbl[])
              n430 = case shown="True" w1046 {
                tunnel: w1048 -> [_ w1090]
                tunnel: w1047 -> [_ w1089]
                frame False {
                }
                frame True {
                  n431 = Subtract(x=w1089, y=299) -> (x-y=w1094:i32)
                  n432 = Index Array(array=w1090, index #1=w1089, index #2=w1094) -> (element #1=w1091:dbl, element #2=w1092:dbl)
                  n433 = Subtract(x=w1091, y=w1092) -> (x-y=→"Addition Rate 1 min. [gr/min]":dbl)
                }
              }
            }
          }
          frame #2 {
            n434 = VISA Close(VISA resource name=w1096, error in (no error)=w1095) -> (error out=w1097:errorcluster)
            n435 = call <vilib>:"Simple Error Handler.vi"("error in (no error)"=w1097) -> ()  [unwired: 1 in, 8 out]
          }
          frame #3 {
            "Peristaltic Balance Restart" <- TRUE ("Peristaltic Balance Restart")
          }
        }
      }
    }
  }
  n436 = while {
    stop <- w1099 stop-if-true
    n437 = property on="Stop Program" class="Bool (strict)"() -> ("Value"=w1099:bool)  [unwired: 2 in, 2 out]
    n438 = Wait (ms)(milliseconds to wait=u32 1000) -> ()  [unwired: 1 out]
    n439 = case shown="True" "Julabo Stainless Steel" {
      frame False {
      }
      frame True {
        n440 = flat-sequence {
          tunnel: [w1111] -> w1106
          tunnel: [w1110] -> w1105
          tunnel: [w1109] -> w1104
          tunnel: w1106 -> [w1141]
          tunnel: w1105 -> [w1140]
          tunnel: w1104 -> [w1139]
          tunnel: [w1138] -> w1103
          tunnel: [w1137] -> w1102
          tunnel: w1103 -> [w1210]
          tunnel: w1102 -> [w1209]
          frame #0 {
            n441 = control-ref of="Boolean 23"() -> (w1113:refnum<vi>)
            n442 = control-ref of="Boolean 24"() -> (w1108:refnum<vi>)
            n443 = control-ref of="Boolean 22"() -> (w1115:refnum<vi>)
            n444 = control-ref of="Boolean 25"() -> (w1116:refnum<vi>)
            n445 = property on="Internal Temp." class="Slide (strict)"("Value"=0.0) -> ()  [unwired: 2 in, 2 out]
            n446 = property on="Julabo SS Restart" class="Bool (strict)"("Value"=FALSE ("Julabo SS Restart")) -> ()  [unwired: 2 in, 2 out]
            n447 = To Unsigned Long Integer(number=4800) -> (unsigned 32bit integer=w1133:u32)
            n448 = To Unsigned Word Integer(number=2) -> (unsigned 16bit integer=w1132:u16)
            n449 = To Unsigned Word Integer(number=7) -> (unsigned 16bit integer=w1126:u16)
            n450 = To Unsigned Word Integer(number=10) -> (unsigned 16bit integer=w1131:u16)
            n451 = To Unsigned Word Integer(number=2) -> (unsigned 16bit integer=w1130:u16)
            n452 = Build Array(w1113, w1108, w1115, w1116) -> (w1117:refnum<vi>[])
            n453 = for {
              tunnel: w1117 -> [w1136] mode=indexing
              tunnel: [w1134] -> w1111 mode=indexing
              n454 = property class="Bool (strict)"(reference=w1136, "Value"=FALSE) -> (reference out=w1134:refnum<vi>)  [unwired: 1 in, 1 out]
            }
            n455 = property on="Start/\nStop" class="Bool (strict)"("Value"=FALSE ("Start/\nStop")) -> ()  [unwired: 2 in, 2 out]
            n456 = Bundle(w1133, w1132, w1126, w1131, w1130) -> (w1129:cluster{u32, u16, u16, u16, u16})  [unwired: 1 in]
            n457 = property on="Set Temp. [°C]" class="DigNum (strict)"("Value"=0.0, "NumText.BGColor"=u32 16711680 ("Numeric Text.Text Colors:BG Color")) -> ()  [unwired: 2 in, 2 out]
            n458 = To Unsigned Long Integer(number=128) -> (unsigned 32bit integer=w1127:u32)
            n459 = call <instrlib>:"Initialize.vi"("RS485-Address (128: RS232)"=w1127, "Serial Configuration"=w1129, "VISA resource name"="Julabo Stainless Steel") -> ("error out"=w1109:errorcluster, "VISA resource name out"=w1110:refnum<visa-resource-name>)  [unwired: 7 in]
          }
          frame #1 {
            n460 = while {
              tunnel: FALSE ("StartStop") -> [w1155]
              tunnel: w1141 -> [w1153]
              tunnel: w1140 -> [w1152]
              tunnel: w1139 -> [w1151]
              tunnel: [w1150] -> w1138
              tunnel: [w1147] -> w1137
              stop <- w1146 stop-if-true
              n461 = Greater?(x="Set Temp. [°C]", y=150.0) -> (0:w1178:bool)
              n462 = Not Equal?(x=w1155, y="Start/\nStop") -> (x != y?=w1166:bool)
              n463 = case shown="False" w1178 {
                tunnel: [w1185 150.0 ("Set Temp.")] -> w1179
                tunnel: "Set Temp. [°C]" -> [w1184 _]
                frame False {
                  n464 = Less?(x=w1184, y=20.0) -> (x < y?=w1187:bool)
                  n465 = case shown="True" w1187 {
                    tunnel: [w1188 20.0 ("y")] -> w1185
                    tunnel: w1184 -> [w1188 _]
                    frame False {
                    }
                    frame True {
                    }
                  }
                }
                frame True {
                }
              }
              n466 = case shown="True" w1166 {
                tunnel: w1151 -> [w1202 w1208]
                tunnel: w1152 -> [w1203 w1207]
                tunnel: [w1201 w1206] -> w1167
                tunnel: [w1200 w1205] -> w1168
                tunnel: "Start/\nStop" -> [w1199 w1204]
                frame False {
                  n467 = call <instrlib>:"StartStop Device.vi"("error in (no error)"=w1202, "Start/Stop (f:Stop)"=w1199, "VISA resource name"=w1203) -> ("error out"=w1201:errorcluster, "VISA resource name out"=w1200:refnum<visa-resource-name>)  [unwired: 7 in]
                }
                frame True {
                  n468 = call <instrlib>:"StartStop Device.vi"("error in (no error)"=w1208, "Start/Stop (f:Stop)"=w1204, "VISA resource name"=w1207) -> ("error out"=w1206:errorcluster, "VISA resource name out"=w1205:refnum<visa-resource-name>)  [unwired: 7 in]
                }
              }
              n469 = call <instrlib>:"Set Setpoint.vi"("Setpointindex (Setpoint1: Default)"=enum16{"Setpoint 1", "Setpoint 2", "Setpoint 3"}."Setpoint 1" ("Setpoint"), "error in (no error)"=w1167, "newSetpoint (20.00°C)"=w1179, "VISA resource name"=w1168) -> ("error out"=w1170:errorcluster, "VISA resource name out"=w1169:refnum<visa-resource-name>)  [unwired: 6 in]
              n470 = property on="Set Temp. [°C]" class="DigNum (strict)"("Value"=w1179) -> ()  [unwired: 2 in, 2 out]
              n471 = Greater?(x="Set Temp. [°C]", y=0.0) -> (0:w1182:bool)
              n472 = call <instrlib>:"Error Handler.vi"("error in (no error)"=w1170, "ClearCommandError (false)"=TRUE, "VISA resource name"=w1169) -> ("error out"=w1165:errorcluster, "VISA resource name out"=w1171:refnum<visa-resource-name>)  [unwired: 5 in, 2 out]
              n473 = case shown="True" w1182 {
                frame False {
                }
                frame True {
                  n474 = property on="Set Temp. [°C]" class="DigNum (strict)"("NumText.BGColor"=u32 65280 ("Numeric Text.Text Colors:BG Color")) -> ()  [unwired: 2 in, 2 out]
                }
              }
              n475 = call <instrlib>:"Get InternalTemp.vi"("error in (no error)"=w1165, "VISA resource name"=w1171) -> ("error out"=w1147:errorcluster, "InternalTemp (out)"=w1180:dbl, "VISA resource name out"=w1150:refnum<visa-resource-name>)  [unwired: 7 in]
              "Internal Temp." <- w1180
              n476 = Subtract(x=150.0, y=w1180) -> (x-y=w1173:dbl)
              n477 = Subtract(x=w1180, y=20.0) -> (x-y=w1174:dbl)
              n478 = Multiply(x=3.1875, y=w1174) -> (x*y=w1175:dbl)
              n479 = Multiply(x=w1173, y=3.1875) -> (x*y=w1176:dbl)
              n480 = call <vilib>:"RGB to Color.vi"("B"=w1176, "G"=u8 0, "R"=w1175) -> ("Color"=w1172:u32)
              n481 = Bundle("Color"=w1172, "Color"=w1172) -> (w1177:cluster{"Color":u32, "Color":u32})  [unwired: 1 in]
              n482 = for {
                tunnel: w1153 -> [w1194] mode=indexing
                tunnel: w1177 -> [w1195]
                n483 = property class="Bool (strict)"(reference=w1194) -> (reference out=w1193:refnum<vi>, "Colors [4]"=→"Colors4":cluster{u32, u32}[])  [unwired: 1 in, 1 out]
                n484 = property on="Colors4" class="Arr (strict)"() -> ("Value"=w1191:cluster{u32, u32}[])  [unwired: 2 in, 2 out]
                n485 = Replace Array Subset(array=w1191, new element=w1195, index=1) -> (w1196:cluster{u32, u32}[])
                n486 = property class="Bool (strict)"(reference=w1193, "Value"=TRUE, "Colors [4]"=w1196) -> ()  [unwired: 1 in, 2 out]
              }
              n487 = property on="Julabo Stainless Steel" class="Bool (strict)"() -> ("Value"=w1145:bool)  [unwired: 2 in, 2 out]
              n488 = property on="Stop Program" class="Bool (strict)"() -> ("Value"=w1144:bool)  [unwired: 2 in, 2 out]
              n489 = Not(x=w1145) -> (.not. x?=w1149:bool)
              n490 = Wait (ms)(milliseconds to wait=u32 1000) -> ()  [unwired: 1 out]
              n491 = Or(x=w1149, y=w1144) -> (x .or. y?=w1148:bool)
              n492 = Or(x=w1148, y=w1147) -> (x .or. y?=w1146:bool)
            }
          }
          frame #2 {
            n493 = call <instrlib>:"Close.vi"("error in (no error)"=w1209, "VISA resource name"=w1210) -> ("error out"=w1211:errorcluster)  [unwired: 9 in]
            n494 = call <vilib>:"Simple Error Handler.vi"("error in (no error)"=w1211) -> ()  [unwired: 4 in, 5 out]
          }
          frame #3 {
            "Julabo SS Restart" <- TRUE ("Julabo SS Restart")
          }
        }
      }
    }
  }
  n495 = flat-sequence {
    tunnel: [w1249] -> w3
    tunnel: w3 -> [w1255]
    frame #0 {
      w1213 = u32 13816530
      n496 = control-ref of="Boolean 33"() -> (w1216:refnum<vi>)
      n497 = control-ref of="Boolean 32"() -> (w1215:refnum<vi>)
      n498 = control-ref of="Boolean 31"() -> (w1228:refnum<vi>)
      n499 = control-ref of="Boolean 27"() -> (w1227:refnum<vi>)
      n500 = control-ref of="Boolean 30"() -> (w1226:refnum<vi>)
      n501 = control-ref of="Boolean"() -> (w1225:refnum<vi>)
      n502 = control-ref of="Boolean 28"() -> (w1224:refnum<vi>)
      n503 = Build Array(w1216, w1215, w1228, w1227, w1226, w1225, w1224) -> (w1229:refnum<vi>[])
      n504 = property on="Seed Time" class="AbsTime (strict)"("Value"=timestamp(0 s since 1904-01-01) ("Seed Time")) -> ()  [unwired: 2 in, 2 out]
      n505 = for {
        tunnel: w1229 -> [w1252] mode=indexing
        tunnel: [w1250] -> w1249 mode=indexing
        n506 = property class="Bool (strict)"(reference=w1252, "Value"=FALSE) -> (reference out=w1250:refnum<vi>)  [unwired: 1 in, 1 out]
      }
      n507 = call-poly <vilib>:"Read Delimited Spreadsheet.vi"("file path (dialog if empty)"=path "C:/Crystallization System/Sucrose Solubility in Impure Sucrose Solutions Bilinear Interpolated Data.txt") -> ("all rows"=→"Interpolated Data":dbl[][])  [unwired: 9 in, 5 out]
      n508 = property on="Torque [Ncm]" class="Str"("Value"="0" ("Torque [Ncm]"), "Text.BGColor"=w1213) -> ()  [unwired: 2 in, 2 out]
      n509 = property on="TS-Mass Graph" class="XYGraph (strict)"("Value"=cluster{dbl[], dbl[]} {[nan, nan, nan, nan, nan, nan, nan, nan, nan, nan, nan, nan, nan, nan, nan, nan, nan, nan, nan, nan, nan, nan, nan, nan, nan, nan, nan, nan, nan, nan, nan, nan, nan, nan, nan, nan, nan, nan, nan, nan, nan, nan, nan, nan, nan, nan, nan, nan, nan, nan, nan, nan, nan, nan, nan, nan, nan, nan, nan, nan, nan, nan, nan, nan, nan, nan, nan, nan, nan, nan, nan, nan, nan, nan, nan, nan, nan], [0.0, 0.0, 0.0, 0.0, 0.0, 0.0, 0.0, 0.0, 0.0, 0.0, 0.0, 0.0, 0.0, 0.0, 0.0, 0.0, 0.0, 0.0, 0.0, 0.0, 0.0, 0.0, 0.0, 0.0, 0.0, 0.0, 0.0, 0.0, 0.0, 0.0, 0.0, 0.0, 0.0, 0.0, 0.0, 0.0, 0.0, 0.0, 0.0, 0.0, 0.0, 0.0, 0.0, 0.0, 0.0, 0.0, 0.0, 0.0, 0.0, 0.0, 0.0, 0.0, 0.0, 0.0, 0.0, 0.0, 0.0, 0.0, 0.0, 0.0, 0.0, 0.0, 0.0, 0.0, 0.0, 0.0, 0.0, 0.0, 0.0, 0.0, 0.0, 0.0, 0.0, 0.0, 0.0, 0.0, 0.0]} ("TS-Mass Graph")) -> ()  [unwired: 2 in, 2 out]
      n510 = property on="Torque [Ncm]" class="Str"("Value"="0" ("Torque [Ncm]"), "Text.BGColor"=w1213) -> ()  [unwired: 2 in, 2 out]
      n511 = property on="Torque [Ncm]" class="Str"("Value"="0" ("Torque [Ncm]"), "Text.BGColor"=w1213) -> ()  [unwired: 2 in, 2 out]
      n512 = property on="dTS&dBX Graph" class="WFChart (strict)"("History Data"=cluster{dbl, "Value":dbl}[] []) -> ()  [unwired: 2 in, 2 out]
      n513 = property on="Supersaturation Graph (Kss)" class="WFChart (strict)"("History Data"=dbl[] []) -> ()  [unwired: 2 in, 2 out]
      n514 = property on="Torque Graph" class="WFChart (strict)"("History Data"=dbl[] []) -> ()  [unwired: 2 in, 2 out]
      n515 = property on="Process 2" class="WFChart (strict)"("History Data"=dbl[] []) -> ()  [unwired: 2 in, 2 out]
      n516 = property on="Elapsed Time" class="DigNum (strict)"("Value"=0.0 ("Elapsed Time")) -> ()  [unwired: 2 in, 2 out]
      n517 = property on="Tank's\nHeight [cm]" class="Slide (strict)"("Value"=0.0 ("Tank's \nVolume [mL]")) -> ()  [unwired: 2 in, 2 out]
      n518 = property on="Tank's Solution\nWeight [gr]" class="Slide (strict)"("Value"=0.0) -> ()  [unwired: 2 in, 2 out]
      n519 = property on="Total Amount Added [gr]" class="DigNum (strict)"("Value"=0.0 ("Amount of Added Syrup [gr]")) -> ()  [unwired: 2 in, 2 out]
      n520 = property on="Amount of Dry Substance\n[gr]" class="DigNum (strict)"("Value"=0.0) -> ()  [unwired: 2 in, 2 out]
      n521 = property on="Amount of Sugar [gr]" class="DigNum (strict)"("Value"=0.0) -> ()  [unwired: 2 in, 2 out]
      n522 = property on="Actual Saturation (Kact)" class="DigNum (strict)"("Value"=0.0) -> ()  [unwired: 2 in, 2 out]
      n523 = property on="Condensate Weight [gr]" class="Slide (strict)"("Value"=0.0) -> ()  [unwired: 2 in, 2 out]
      n524 = property on="°Bx" class="DigNum (strict)"("Value"=0.0) -> ()  [unwired: 2 in, 2 out]
      n525 = property on="Dry Substance [%]" class="Slide (strict)"("Value"=0.0) -> ()  [unwired: 2 in, 2 out]
      n526 = property on="Sugar [%]" class="Slide (strict)"("Value"=0.0) -> ()  [unwired: 2 in, 2 out]
      n527 = property on="Saturation (Ks)" class="DigNum (strict)"("Value"=0.0) -> ()  [unwired: 2 in, 2 out]
      n528 = property on="Supersaturation (Kss)" class="DigNum (strict)"("Value"=0.0) -> ()  [unwired: 2 in, 2 out]
      n529 = property on="Temp. [°C]" class="DigNum (strict)"("Value"=0.0 ("Temp. [°C]")) -> ()  [unwired: 2 in, 2 out]
      n530 = property on="Temp. [°C]" class="DigNum (strict)"("Value"=0.0) -> ()  [unwired: 2 in, 2 out]
      n531 = property on="Table Value" class="DigNum (strict)"("Value"=0.0) -> ()  [unwired: 2 in, 2 out]
    }
    frame #1 {
      n532 = while {
        shift-right: [w1269] -> _
        shift-left: 0.0 -> [w1307]
        shift-right: [w1271] -> _
        shift-left: 0.0 -> [w1306]
        shift-right: [w1270] -> _
        shift-left: 0.0 -> [w1316]
        tunnel: w1255 -> [w1284]
        shift-right: [w1265] -> _
        shift-left: dbl[] [] -> [w1267]
        shift-right: [w1264] -> _
        shift-left: dbl[] [] -> [w1266]
        i -> [w1274]
        stop <- "Stop Program" stop-if-true
        n533 = case shown="True" "Add Syrup" {
          tunnel: w1316 -> [w1407 w1427]
          tunnel: [w1407 w1415] -> w1294
          tunnel: w1307 -> [w1406 w1425]
          tunnel: [w1406 w1424] -> w1296
          tunnel: w1306 -> [w1405 w1422]
          tunnel: [w1405 w1416] -> w1295
          tunnel: w1284 -> [w1404 w1414]
          frame False {
            n534 = property on="Pipe Delay" class="DigNum (strict)"() -> ("Value"=w1398:dbl)  [unwired: 2 in, 2 out]
            n535 = property on="Boolean 31" class="Bool (strict)"() -> ("Value"=w1402:bool)  [unwired: 2 in, 2 out]
            n536 = Add(x=w1398, y=1.0) -> (x+y=w1399:dbl)
            n537 = Greater?(x=w1398, y=5.0) -> (0:w1401:bool)
            n538 = property on="Pipe Delay" class="DigNum (strict)"("Value"=w1399) -> ()  [unwired: 2 in, 2 out]
            n539 = And(x=w1402, y=w1401) -> (x .and. y?=w1397:bool)
            n540 = case shown="False" w1397 {
              tunnel: w1404 -> [_ w1409]
              frame False {
              }
              frame True {
                n541 = for {
                  tunnel: w1409 -> [w1412] mode=indexing
                  tunnel: [w1410] -> _ mode=indexing
                  n542 = property class="Bool (strict)"(reference=w1412, "Value"=FALSE) -> (reference out=w1410:refnum<vi>)  [unwired: 1 in, 1 out]
                }
              }
            }
            n543 = case shown="False" w1397 {
              frame False {
              }
              frame True {
                "Pipe Delay" <- 0.0 ("Pipe Delay")
              }
            }
          }
          frame True {
            n544 = flat-sequence {
              tunnel: w1425 -> [w1434]
              tunnel: [w1433] -> w1426
              tunnel: ["Syrup Addition [gr]"] -> w1423
              tunnel: [w1436] -> w1424
              tunnel: w1426 -> [w1436]
              frame #0 {
                n545 = Add(x=w1434, y="Syrup Addition [gr]") -> (x+y=w1433:dbl)
              }
              frame #1 {
                n546 = property on="Syrup Addition [gr]" class="Slide (strict)"("Value"=0.0) -> ()  [unwired: 2 in, 2 out]
                "Total Amount Added [gr]" <- w1436
              }
            }
            n547 = for {
              tunnel: w1414 -> [w1431] mode=indexing
              tunnel: [w1429] -> _ mode=indexing
              n548 = property class="Bool (strict)"(reference=w1431, "Value"=TRUE) -> (reference out=w1429:refnum<vi>)  [unwired: 1 in, 1 out]
            }
            n549 = Divide(x="°Bx In-Line", y=100.0) -> (x/y=w1419:dbl)
            n550 = Multiply(x=w1423, y=w1419) -> (x*y=w1421:dbl)
            n551 = Multiply(x=w1421, y="Purity (0.92-1.0)") -> (x*y=w1428:dbl)
            n552 = Add(x=w1428, y=w1427) -> (x+y=w1415:dbl)
            "Amount of Sugar [gr]" <- w1415
            n553 = Add(x=w1421, y=w1422) -> (x+y=w1416:dbl)
            "Amount of Dry Substance\n[gr]" <- w1416
            n554 = property on="Pipe Delay" class="DigNum (strict)"("Value"=0.0 ("Pipe Delay")) -> ()  [unwired: 2 in, 2 out]
          }
        }
        n555 = flat-sequence {
          tunnel: [w1361] -> w1299
          frame #0 {
            n556 = call <vilib>:"System Exec.vi"("run minimized? (F)"=TRUE, "command line"="C:\\Program Files (x86)\\QTenki\\usbtenkiget.exe -s E14591 -i 0") -> ("standard output"=w1355:string)  [unwired: 6 in, 3 out]
            n557 = Fract/Exp String To Number(string=w1355) -> (number=→"Temp. [°C]":dbl)  [unwired: 3 in, 1 out]
          }
          frame #1 {
            n558 = property on="Amount of Sugar [gr]" class="DigNum (strict)"() -> ("Value"=w1357:dbl)  [unwired: 2 in, 2 out]
            n559 = property on="Amount of Dry Substance\n[gr]" class="DigNum (strict)"() -> ("Value"=w1356:dbl)  [unwired: 2 in, 2 out]
            n560 = Divide(x=w1357, y=w1356) -> (x/y=w1358:dbl)
            n561 = property on="Temp. [°C]" class="DigNum (strict)"() -> ("Value"=w1362:dbl)  [unwired: 2 in, 2 out]
            n562 = Greater Or Equal?(x=w1358, y=0.92) -> (x >= y?=w1364:bool)
            n563 = Less Or Equal?(x=w1362, y=90.0) -> (x <= y?=w1363:bool)
            n564 = Multiply(x=100.0, y=w1358) -> (x*y=w1360:dbl)
            n565 = And(x=w1364, y=w1363) -> (x .and. y?=w1365:bool)
            n566 = case shown="True" w1365 {
              tunnel: w1360 -> [_ w1370]
              tunnel: w1362 -> [_ w1371]
              tunnel: [-1.0 ("Numeric") w1369] -> w1361
              frame False {
              }
              frame True {
                n567 = property on="Interpolated Data" class="Arr (strict)"() -> ("Value"=w1372:dbl[][])  [unwired: 2 in, 2 out]
                n568 = Subtract(x=w1371, y=20.0) -> (x-y=w1377:dbl)
                n569 = Subtract(x=w1370, y=92.0) -> (x-y=w1378:dbl)
                n570 = Multiply(x=100.0, y=w1377) -> (x*y=w1379:dbl)
                n571 = Multiply(x=100.0, y=w1378) -> (x*y=w1380:dbl)
                n572 = Index Array(array=w1372, index (row)=w1380, index (col)=w1379) -> (element=w1369:dbl)
                "Table Value" <- w1369
              }
            }
          }
        }
        n573 = property on="Start/Stop" class="Bool (strict)"() -> ("Value"=w1297:bool)  [unwired: 2 in, 2 out]
        n574 = case shown="True" w1297 {
          tunnel: w1296 -> [w1383 w1391]
          tunnel: w1295 -> [w1381 w1388]
          tunnel: w1294 -> [w1382 w1386]
          tunnel: [w1383 w1391] -> w1280
          tunnel: [w1382 w1386] -> w1282
          tunnel: [w1381 w1388] -> w1281
          frame False {
          }
          frame True {
            n575 = property on="Syrup Added [gr]" class="Slide (strict)"() -> ("Value"=w1390:dbl)  [unwired: 2 in, 2 out]
            n576 = Divide(x="Dry Substance [%]", y=100.0) -> (x/y=w1395:dbl)
            n577 = Multiply(x=w1390, y=w1395) -> (x*y=w1389:dbl)
            n578 = Add(x=w1391, y=w1390) -> (x+y=w1392:dbl)
            n579 = Multiply(x=w1389, y="Purity (0.92-1.0)") -> (x*y=w1387:dbl)
            n580 = Add(x=w1388, y=w1389) -> (x+y=w1394:dbl)
            n581 = Add(x=w1386, y=w1387) -> (x+y=w1393:dbl)
            n582 = property on="Total Amount Added [gr]" class="DigNum (strict)"("Value"=w1392) -> ()  [unwired: 2 in, 2 out]
            n583 = property on="Amount of Dry Substance\n[gr]" class="DigNum (strict)"("Value"=w1394) -> ()  [unwired: 2 in, 2 out]
            n584 = property on="Amount of Sugar [gr]" class="DigNum (strict)"("Value"=w1393) -> ()  [unwired: 2 in, 2 out]
          }
        }
        n585 = case shown="True" "Add Seeds" {
          tunnel: w1282 -> [w1334 w1349]
          tunnel: w1281 -> [w1336 w1351]
          tunnel: [w1336 w1350] -> w1271
          tunnel: w1280 -> [w1335 w1346]
          tunnel: [w1335 w1345] -> w1269
          tunnel: [w1334 w1348] -> w1270
          frame False {
          }
          frame True {
            n586 = property on="Seeds Added" class="Bool (strict)"("Value"=TRUE ("Seeds Added")) -> ()  [unwired: 2 in, 2 out]
            n587 = Add(x="Amount [gr]", y=w1349) -> (x+y=w1348:dbl)
            n588 = Add(x=w1346, y="Amount [gr]") -> (x+y=w1345:dbl)
            n589 = Add(x="Amount [gr]", y=w1351) -> (x+y=w1350:dbl)
            n590 = property on="Total Amount Added [gr]" class="DigNum (strict)"("Value"=w1345) -> ()  [unwired: 2 in, 2 out]
            n591 = property on="Amount of Dry Substance\n[gr]" class="DigNum (strict)"("Value"=w1350) -> ()  [unwired: 2 in, 2 out]
            n592 = property on="Amount of Sugar [gr]" class="DigNum (strict)"("Value"=w1348) -> ()  [unwired: 2 in, 2 out]
            n593 = property on="Supersaturation (Kss)" class="DigNum (strict)"() -> ("Value"=→"Seeding Kss":dbl)  [unwired: 2 in, 2 out]
            n594 = property on="°Bx" class="DigNum (strict)"() -> ("Value"=→"Seeding °Bx":dbl)  [unwired: 2 in, 2 out]
            n595 = property on="Internal Temp." class="Slide (strict)"() -> ("Value"=→"Seeding Julabo Glass Temp. [°C]":dbl)  [unwired: 2 in, 2 out]
            n596 = property on="Internal Temp." class="Slide (strict)"() -> ("Value"=→"Seeding Julabo SS Temp. [°C]":dbl)  [unwired: 2 in, 2 out]
            n597 = property on="Set Speed RPM" class="DigNum (strict)"() -> ("Value"=→"Seeding RPM":dbl)  [unwired: 2 in, 2 out]
            n598 = property on="Temp. [°C]" class="DigNum (strict)"() -> ("Value"=→"Seeding Temp. [°C]":dbl)  [unwired: 2 in, 2 out]
            n599 = Get Date/Time In Seconds() -> (seconds since 1Jan1904=→"Seed Time":timestamp)
          }
        }
        n600 = property on="Amount of Dry Substance\n[gr]" class="DigNum (strict)"() -> ("Value"=w1260:dbl)  [unwired: 2 in, 2 out]
        n601 = property on="Amount of Sugar [gr]" class="DigNum (strict)"() -> ("Value"=w1259:dbl)  [unwired: 2 in, 2 out]
        n602 = property on="°Bx" class="DigNum (strict)"() -> ("Value"=w1298:dbl)  [unwired: 2 in, 2 out]
        "Dry Substance [%]" <- w1298
        n603 = property on="Total Amount Added [gr]" class="DigNum (strict)"() -> ("Value"=w1261:dbl)  [unwired: 2 in, 2 out]
        n604 = property on="Condensate Weight [gr]" class="Slide (strict)"() -> ("Value"=w1305:dbl)  [unwired: 2 in, 2 out]
        n605 = Divide(x=w1259, y=w1260) -> (x/y=w1313:dbl)
        n606 = property on="Seeds Added" class="Bool (strict)"() -> ("Value"=w1263:bool)  [unwired: 2 in, 2 out]
        n607 = Multiply(x=w1313, y=w1298) -> (x*y=w1303:dbl)
        "Sugar [%]" <- w1303
        n608 = Subtract(x=w1261, y=w1305) -> (x-y=w1268:dbl)
        "Tank's Solution\nWeight [gr]" <- w1268
        n609 = Divide(x=w1260, y=w1268) -> (x/y=w1315:dbl)
        n610 = Subtract(x=100.0 ("y"), y=w1298) -> (x-y=w1312:dbl)
        n611 = Add(x=1 ("y"), y=w1274) -> (x+y=w1279:i32)
        n612 = Multiply(x=w1315, y=100.0) -> (x*y=w1262:dbl)
        "Dry Substance [%]" <- w1262
        n613 = case shown="True" w1263 {
          tunnel: w1262 -> [_ w1332]
          tunnel: w1268 -> [_ w1331]
          tunnel: [w1317 w1327] -> w1264
          tunnel: [w1318 w1326] -> w1265
          tunnel: w1267 -> [w1318 w1330]
          tunnel: w1266 -> [w1317 w1329]
          frame False {
          }
          frame True {
            n614 = Get Date/Time In Seconds() -> (seconds since 1Jan1904=w1325:timestamp)
            n615 = property on="Seed Time" class="AbsTime (strict)"() -> ("Value"=w1323:timestamp)  [unwired: 2 in, 2 out]
            n616 = To Double Precision Float(number=w1325) -> (double precision float=w1324:dbl)
            n617 = To Double Precision Float(number=w1323) -> (double precision float=w1322:dbl)
            n618 = Build Array (concatenate)(w1330, w1331) -> (w1326:dbl[])
            n619 = Subtract(x=w1324, y=w1322) -> (x-y=w1321:dbl)
            n620 = Build Array (concatenate)(w1329, w1332) -> (w1327:dbl[])
            n621 = Divide(x=w1321, y=60.0) -> (x/y=→"Elapsed Time":dbl)
            n622 = Bundle(w1327, w1326) -> (→"TS-Mass Graph":cluster{dbl[], dbl[]})  [unwired: 1 in]
          }
        }
        n623 = Divide(x=w1303, y=w1312) -> (x/y=w1302:dbl)
        "Actual Saturation (Kact)" <- w1302
        n624 = Subtract(x=100.0 ("y"), y=w1303) -> (x-y=w1308:dbl)
        n625 = Quotient & Remainder(x=w1279, y=30) -> (x-y*floor(x/y)=w1277:i32)  [unwired: 1 out]
        n626 = Divide(x=w1302, y=w1299) -> (x/y=w1273:dbl)
        "Supersaturation (Kss)" <- w1273
        n627 = Equal?(x=0, y=w1277) -> (x = y?=w1272:bool)
        n628 = Divide(x=w1268, y=1.313) -> (x/y=w1285:dbl)
        n629 = Divide(x=w1303, y=w1308) -> (x/y=→"Saturation (Ks)":dbl)
        n630 = Divide(x=13.0 ("y"), y=2.0) -> (x/y=w1289:dbl)
        n631 = case shown="True" w1272 {
          tunnel: w1273 -> [_ w1333]
          frame False {
          }
          frame True {
            "Supersaturation Graph (Kss)" <- w1333
          }
        }
        n632 = Square(x=w1289) -> (x^2=w1288:dbl)
        n633 = Wait (ms)(milliseconds to wait=u32 1000) -> ()  [unwired: 1 out]
        n634 = Multiply(x=3.141592653589793, y=w1288) -> (x*y=w1286:dbl)
        n635 = Divide(x=w1285, y=w1286) -> (x/y=→"Tank's\nHeight [cm]":dbl)
      }
    }
  }
  n636 = while {
    stop <- w1437 stop-if-true
    n637 = property on="Stop Program" class="Bool (strict)"() -> ("Value"=w1437:bool)  [unwired: 2 in, 2 out]
    n638 = Wait (ms)(milliseconds to wait=u32 1000) -> ()  [unwired: 1 out]
    n639 = case shown="True" "Julabo Glass" {
      frame False {
      }
      frame True {
        n640 = flat-sequence {
          tunnel: [w1449] -> w1444
          tunnel: [w1448] -> w1443
          tunnel: [w1447] -> w1442
          tunnel: w1444 -> [w1479]
          tunnel: w1443 -> [w1478]
          tunnel: w1442 -> [w1477]
          tunnel: [w1476] -> w1441
          tunnel: [w1475] -> w1440
          tunnel: w1441 -> [w1548]
          tunnel: w1440 -> [w1547]
          frame #0 {
            n641 = control-ref of="Boolean 18"() -> (w1455:refnum<vi>)
            n642 = control-ref of="Boolean 21"() -> (w1454:refnum<vi>)
            n643 = control-ref of="Boolean 19"() -> (w1452:refnum<vi>)
            n644 = control-ref of="Boolean 20"() -> (w1453:refnum<vi>)
            n645 = property on="Internal Temp." class="Slide (strict)"("Value"=0.0) -> ()  [unwired: 2 in, 2 out]
            n646 = property on="Julabo Glass Restart" class="Bool (strict)"("Value"=FALSE ("Julabo Circulators Restart")) -> ()  [unwired: 2 in, 2 out]
            n647 = To Unsigned Long Integer(number=4800) -> (unsigned 32bit integer=w1471:u32)
            n648 = To Unsigned Word Integer(number=2) -> (unsigned 16bit integer=w1470:u16)
            n649 = To Unsigned Word Integer(number=7) -> (unsigned 16bit integer=w1464:u16)
            n650 = To Unsigned Word Integer(number=10) -> (unsigned 16bit integer=w1469:u16)
            n651 = To Unsigned Word Integer(number=2) -> (unsigned 16bit integer=w1468:u16)
            n652 = Build Array(w1455, w1454, w1452, w1453) -> (w1456:refnum<vi>[])
            n653 = for {
              tunnel: w1456 -> [w1474] mode=indexing
              tunnel: [w1472] -> w1447 mode=indexing
              n654 = property class="Bool (strict)"(reference=w1474, "Value"=FALSE) -> (reference out=w1472:refnum<vi>)  [unwired: 1 in, 1 out]
            }
            n655 = Bundle(w1471, w1470, w1464, w1469, w1468) -> (w1467:cluster{u32, u16, u16, u16, u16})  [unwired: 1 in]
            n656 = property on="Set Temp. [°C]" class="DigNum (strict)"("Value"=0.0, "NumText.BGColor"=u32 16711680 ("Numeric Text.Text Colors:BG Color")) -> ()  [unwired: 2 in, 2 out]
            n657 = property on="Start/\nStop" class="Bool (strict)"("Value"=FALSE ("Start/\nStop")) -> ()  [unwired: 2 in, 2 out]
            n658 = To Unsigned Long Integer(number=128) -> (unsigned 32bit integer=w1465:u32)
            n659 = call <instrlib>:"Initialize.vi"("RS485-Address (128: RS232)"=w1465, "Serial Configuration"=w1467, "VISA resource name"="Julabo Glass") -> ("error out"=w1448:errorcluster, "VISA resource name out"=w1449:refnum<visa-resource-name>)  [unwired: 7 in]
          }
          frame #1 {
            n660 = while {
              tunnel: FALSE ("StartStop") -> [w1488]
              tunnel: w1479 -> [w1485]
              tunnel: w1478 -> [w1484]
              tunnel: w1477 -> [w1483]
              tunnel: [w1482] -> w1476
              tunnel: [w1481] -> w1475
              stop <- w1486 stop-if-true
              n661 = Greater?(x="Set Temp. [°C]", y=150.0) -> (0:w1516:bool)
              n662 = Not Equal?(x="Start/\nStop", y=w1488) -> (x != y?=w1498:bool)
              n663 = case shown="False" w1516 {
                tunnel: [w1523 150.0 ("Set Temp.")] -> w1517
                tunnel: "Set Temp. [°C]" -> [w1522 _]
                frame False {
                  n664 = Less?(x=w1522, y=20.0) -> (x < y?=w1525:bool)
                  n665 = case shown="True" w1525 {
                    tunnel: [w1526 20.0 ("y")] -> w1523
                    tunnel: w1522 -> [w1526 _]
                    frame False {
                    }
                    frame True {
                    }
                  }
                }
                frame True {
                }
              }
              n666 = case shown="True" w1498 {
                tunnel: w1484 -> [w1540 w1546]
                tunnel: w1485 -> [w1541 w1545]
                tunnel: [w1539 w1543] -> w1499
                tunnel: [w1538 w1544] -> w1500
                tunnel: "Start/\nStop" -> [w1537 w1542]
                frame False {
                  n667 = call <instrlib>:"StartStop Device.vi"("error in (no error)"=w1540, "Start/Stop (f:Stop)"=w1537, "VISA resource name"=w1541) -> ("error out"=w1538:errorcluster, "VISA resource name out"=w1539:refnum<visa-resource-name>)  [unwired: 7 in]
                }
                frame True {
                  n668 = call <instrlib>:"StartStop Device.vi"("error in (no error)"=w1546, "Start/Stop (f:Stop)"=w1542, "VISA resource name"=w1545) -> ("error out"=w1544:errorcluster, "VISA resource name out"=w1543:refnum<visa-resource-name>)  [unwired: 7 in]
                }
              }
              n669 = call <instrlib>:"Set Setpoint.vi"("Setpointindex (Setpoint1: Default)"=enum16{"Setpoint 1", "Setpoint 2", "Setpoint 3"}."Setpoint 1" ("Setpoint"), "error in (no error)"=w1500, "newSetpoint (20.00°C)"=w1517, "VISA resource name"=w1499) -> ("error out"=w1502:errorcluster, "VISA resource name out"=w1501:refnum<visa-resource-name>)  [unwired: 6 in]
              n670 = property on="Set Temp. [°C]" class="DigNum (strict)"("Value"=w1517) -> ()  [unwired: 2 in, 2 out]
              n671 = call <instrlib>:"Error Handler.vi"("error in (no error)"=w1502, "ClearCommandError (false)"=TRUE, "VISA resource name"=w1501) -> ("error out"=w1504:errorcluster, "VISA resource name out"=w1503:refnum<visa-resource-name>)  [unwired: 5 in, 2 out]
              n672 = call <instrlib>:"Get InternalTemp.vi"("error in (no error)"=w1504, "VISA resource name"=w1503) -> ("error out"=w1481:errorcluster, "InternalTemp (out)"=w1518:dbl, "VISA resource name out"=w1482:refnum<visa-resource-name>)  [unwired: 7 in]
              "Internal Temp." <- w1518
              n673 = Subtract(x=150.0, y=w1518) -> (x-y=w1511:dbl)
              n674 = Subtract(x=w1518, y=20.0) -> (x-y=w1512:dbl)
              n675 = Multiply(x=3.1875, y=w1512) -> (x*y=w1513:dbl)
              n676 = Multiply(x=w1511, y=3.1875) -> (x*y=w1514:dbl)
              n677 = call <vilib>:"RGB to Color.vi"("B"=w1514, "G"=u8 0, "R"=w1513) -> ("Color"=w1515:u32)
              n678 = Bundle("Color"=w1515, "Color"=w1515) -> (w1510:cluster{"Color":u32, "Color":u32})  [unwired: 1 in]
              n679 = Greater?(x="Set Temp. [°C]", y=0.0) -> (0:w1520:bool)
              n680 = for {
                tunnel: w1483 -> [w1532] mode=indexing
                tunnel: w1510 -> [w1533]
                n681 = property class="Bool (strict)"(reference=w1532) -> (reference out=w1531:refnum<vi>, "Colors [4]"=w1530:cluster{u32, u32}[])  [unwired: 1 in, 1 out]
                n682 = property on="Colors4" class="Arr (strict)"("Value"=w1530) -> ()  [unwired: 2 in, 2 out]
                n683 = property on="Colors4" class="Arr (strict)"() -> ("Value"=w1529:cluster{u32, u32}[])  [unwired: 2 in, 2 out]
                n684 = Replace Array Subset(array=w1529, new element=w1533, index=1) -> (w1534:cluster{u32, u32}[])
                n685 = property class="Bool (strict)"(reference=w1531, "Value"=TRUE, "Colors [4]"=w1534) -> ()  [unwired: 1 in, 2 out]
              }
              n686 = case shown="True" w1520 {
                frame False {
                }
                frame True {
                  n687 = property on="Set Temp. [°C]" class="DigNum (strict)"("NumText.BGColor"=u32 65280 ("Numeric Text.Text Colors:BG Color")) -> ()  [unwired: 2 in, 2 out]
                }
              }
              n688 = property on="Julabo Glass" class="Bool (strict)"() -> ("Value"=w1508:bool)  [unwired: 2 in, 2 out]
              n689 = property on="Stop Program" class="Bool (strict)"() -> ("Value"=w1505:bool)  [unwired: 2 in, 2 out]
              n690 = Wait (ms)(milliseconds to wait=u32 1000) -> ()  [unwired: 1 out]
              n691 = Not(x=w1508) -> (.not. x?=w1509:bool)
              n692 = Or(x=w1509, y=w1505) -> (x .or. y?=w1506:bool)
              n693 = Or(x=w1506, y=w1481) -> (x .or. y?=w1486:bool)
            }
          }
          frame #2 {
            n694 = call <instrlib>:"Close.vi"("error in (no error)"=w1547, "VISA resource name"=w1548) -> ("error out"=w1549:errorcluster)  [unwired: 9 in]
            n695 = call <vilib>:"Simple Error Handler.vi"("error in (no error)"=w1549) -> ()  [unwired: 4 in, 5 out]
          }
          frame #3 {
            "Julabo Glass Restart" <- TRUE ("Julabo Circulators Restart")
          }
        }
      }
    }
  }
  n696 = flat-sequence {
    frame #0 {
      n697 = property on="Temp. [°C] by PT100" class="DigNum (strict)"("Value"=0.0 ("Temp. [°C] by PT100")) -> ()  [unwired: 2 in, 2 out]
      n698 = property on="Tank's Height [cm]" class="DigNum (strict)"("Value"=0.0 ("Tank's Height [cm]")) -> ()  [unwired: 2 in, 2 out]
      n699 = property on="Condensate Weight [gr]" class="DigNum (strict)"("Value"=0.0 ("Condensate Weight [gr]")) -> ()  [unwired: 2 in, 2 out]
      n700 = property on="Syrup Added [gr]" class="DigNum (strict)"("Value"=0.0 ("Supersaturation (Kss)")) -> ()  [unwired: 2 in, 2 out]
      n701 = property on="Total Solids (TS)" class="DigNum (strict)"("Value"=0.0 ("Total Solids (TS)")) -> ()  [unwired: 2 in, 2 out]
      n702 = property on="°Bx" class="DigNum (strict)"("Value"=0.0 ("°Bx")) -> ()  [unwired: 2 in, 2 out]
      n703 = property on="Temp. [°C] by RF" class="DigNum (strict)"("Value"=0.0 ("Temp. [°C] by RF")) -> ()  [unwired: 2 in, 2 out]
      n704 = property on="Update Time" class="Str"("Value"="" ("Update Time")) -> ()  [unwired: 2 in, 2 out]
      n705 = property on="Seeds Added" class="Bool (strict)"("Value"=FALSE ("Seeds Added")) -> ()  [unwired: 2 in, 2 out]
    }
    frame #1 {
      n706 = while {
        stop <- w1562 stop-if-true
        n707 = property on="Stop Program" class="Bool (strict)"() -> ("Value"=w1562:bool)  [unwired: 2 in, 2 out]
        n708 = property on="Seeds Added" class="Bool (strict)"() -> ("Value"=w1560:bool)  [unwired: 2 in, 2 out]
        n709 = Wait (ms)(milliseconds to wait=1000) -> ()  [unwired: 1 out]
        n710 = case shown="True" w1560 {
          frame False {
          }
          frame True {
            n711 = while {
              shift-right: [w1569] -> w1564
              shift-left: errorcluster {"status"=FALSE, "code"=0, "source"=""} ("error out") -> [w1573]
              shift-right: [300] -> _
              shift-left: 0 -> [w1567]
              stop <- w1571 stop-if-true
              n712 = call "Elapsed Time"("Time Target (s)"=w1567, "Auto Reset"=TRUE, "error in (no error)"=w1573) -> ("Time has Elapsed"=w1568:bool, "error out"=w1572:errorcluster)  [unwired: 9 in, 6 out]
              n713 = case shown="True" w1568 {
                tunnel: w1572 -> [w1576 w1588]
                tunnel: [w1576 w1588] -> w1569
                frame False {
                }
                frame True {
                  n714 = property on="Condensate Weight [gr]" class="Slide (strict)"() -> ("Value"=→"Condensate Weight [gr]":dbl)  [unwired: 2 in, 2 out]
                  n715 = property on="Syrup Added [gr]" class="Slide (strict)"() -> ("Value"=→"Syrup Added [gr]":dbl)  [unwired: 2 in, 2 out]
                  n716 = property on="Torque [Ncm]" class="Str"() -> ("Value"=→"Torque [Ncm]":string)  [unwired: 2 in, 2 out]
                  n717 = property on="°Bx" class="DigNum (strict)"() -> ("Value"=→"°Bx":dbl)  [unwired: 2 in, 2 out]
                  n718 = property on="Temp. [°C]" class="DigNum (strict)"() -> ("Value"=→"Temp. [°C] by RF":dbl)  [unwired: 2 in, 2 out]
                  n719 = property on="Tank's\nHeight [cm]" class="Slide (strict)"() -> ("Value"=→"Tank's Height [cm]":dbl)  [unwired: 2 in, 2 out]
                  n720 = property on="Dry Substance [%]" class="Slide (strict)"() -> ("Value"=→"Total Solids (TS)":dbl)  [unwired: 2 in, 2 out]
                  n721 = property on="Temp. [°C]" class="DigNum (strict)"() -> ("Value"=→"Temp. [°C] by PT100":dbl)  [unwired: 2 in, 2 out]
                  n722 = Get Date/Time In Seconds() -> (seconds since 1Jan1904=w1582:timestamp)
                  n723 = Format Date/Time String(time format string (%c)="%H:%M:%S", seconds (now)=w1582) -> (date/time string=→"Update Time":string)  [unwired: 1 in]
                }
              }
              n724 = property on="Stop Program" class="Bool (strict)"() -> ("Value"=w1570:bool)  [unwired: 2 in, 2 out]
              n725 = Wait (ms)(milliseconds to wait=u32 100) -> ()  [unwired: 1 out]
              n726 = Or(x=w1569, y=w1570) -> (x .or. y?=w1571:bool)
            }
            n727 = call <vilib>:"Simple Error Handler.vi"("error in (no error)"=w1564) -> ()  [unwired: 4 in, 5 out]
          }
        }
      }
    }
  }
  n728 = flat-sequence {
    tunnel: [w1620] -> w2
    tunnel: [w1618] -> w1
    tunnel: w2 -> [w1640]
    tunnel: w1 -> [w1639]
    frame #0 {
      n729 = control-ref of="Cent. Duration (MM:SS)"() -> (w1595:refnum<vi>)
      n730 = control-ref of="°Bx DM"() -> (w1600:refnum<vi>)
      n731 = control-ref of="Syrup Addition [gr]"() -> (w1592:refnum<vi>)
      n732 = control-ref of="Amount [gr]"() -> (w1617:refnum<vi>)
      n733 = control-ref of="Purity (0.92-1.0)"() -> (w1630:refnum<vi>)
      n734 = control-ref of="°Bx In-Line"() -> (w1621:refnum<vi>)
      n735 = control-ref of="Percentage [%]"() -> (w1608:refnum<vi>)
      n736 = control-ref of="Speed"() -> (w1594:refnum<vi>)
      n737 = control-ref of="Speed RPM"() -> (w1609:refnum<vi>)
      n738 = control-ref of="pH"() -> (w1610:refnum<vi>)
      n739 = control-ref of="Yield [%]"() -> (w1622:refnum<vi>)
      n740 = control-ref of="Emptying 2nd\nCycle [gr]"() -> (w1623:refnum<vi>)
      n741 = control-ref of="Emptying 1st\nCycle [gr]"() -> (w1624:refnum<vi>)
      n742 = control-ref of="Feed 2nd Cycle [gr]"() -> (w1625:refnum<vi>)
      n743 = control-ref of="Feed 1st Cycle [gr]"() -> (w1626:refnum<vi>)
      n744 = control-ref of="Loading 2nd\nCycle [gr]"() -> (w1627:refnum<vi>)
      n745 = control-ref of="Loading 1st\nCycle [gr]"() -> (w1628:refnum<vi>)
      n746 = control-ref of="Silverson Duration (MM:SS)"() -> (w1593:refnum<vi>)
      n747 = control-ref of="Syrup °Bx by Manual RF"() -> (w1591:refnum<vi>)
      n748 = control-ref of="Sugar Source"() -> (w1607:refnum<vi>)
      n749 = control-ref of="Comments"() -> (w1606:refnum<vi>)
      n750 = control-ref of="Additives"() -> (w1605:refnum<vi>)
      n751 = control-ref of="Size (um)"() -> (w1614:refnum<vi>)
      n752 = control-ref of="Method"() -> (w1615:refnum<vi>)
      n753 = control-ref of="Seed Type"() -> (w1616:refnum<vi>)
      n754 = control-ref of="Experiment Name"() -> (w1613:refnum<vi>)
      n755 = control-ref of="Experiment Type"() -> (w1612:refnum<vi>)
      n756 = control-ref of="Operator Name"() -> (w1611:refnum<vi>)
      n757 = Build Array(w1595, w1600, w1592, w1617, w1630, w1621, w1608, w1594, w1609, w1610, w1622, w1623, w1624, w1625, w1626, w1627, w1628, w1593, w1591) -> (w1629:refnum<vi>[])
      n758 = for {
        tunnel: w1629 -> [w1638] mode=indexing
        tunnel: [w1637] -> w1620 mode=indexing
        n759 = property class="DigNum (strict)"(reference=w1638, "Value"=0.0 ("Tank's \nVolume [mL]"), "NumText.BGColor"=u32 16711680 ("Numeric Text.Text Colors:BG Color")) -> (reference out=w1637:refnum<vi>)  [unwired: 1 in, 1 out]
      }
      n760 = property on="Mixing RPM" class="DigNum (strict)"("Value"=900.0 ("Time Interval"), "NumText.BGColor"=u32 16711680 ("Numeric Text.Text Colors:BG Color")) -> ()  [unwired: 2 in, 2 out]
      n761 = property on="Loading Delay" class="AbsTime (strict)"("Value"=timestamp(-7191 s since 1904-01-01) ("Syrup Preparation Time"), "NumText.BGColor"=u32 16711680 ("Numeric Text.Text Colors:BG Color")) -> ()  [unwired: 2 in, 2 out]
      n762 = property on="Time Interval" class="DigNum (strict)"("Value"=30.0 ("Time Interval"), "NumText.BGColor"=u32 16711680 ("Numeric Text.Text Colors:BG Color")) -> ()  [unwired: 2 in, 2 out]
      n763 = Build Array(w1607, w1606, w1605, w1614, w1615, w1616, w1613, w1612, w1611) -> (w1619:refnum<vi>[])
      n764 = for {
        tunnel: w1619 -> [w1634] mode=indexing
        tunnel: [w1633] -> w1618 mode=indexing
        n765 = property class="Str"(reference=w1634, "Value"="", "Text.BGColor"=u32 16711680 ("Numeric Text.Text Colors:BG Color")) -> (reference out=w1633:refnum<vi>)  [unwired: 1 in, 1 out]
      }
      n766 = property on="Temp. [°C]" class="DigNum (strict)"("Value"=70.0, "NumText.BGColor"=u32 16711680 ("Numeric Text.Text Colors:BG Color")) -> ()  [unwired: 2 in, 2 out]
      n767 = property on="Mixing Time" class="DigNum (strict)"("Value"=1200.0 ("Mixing Time"), "NumText.BGColor"=u32 16711680 ("Numeric Text.Text Colors:BG Color")) -> ()  [unwired: 2 in, 2 out]
    }
    frame #1 {
      n768 = while {
        tunnel: w1640 -> [w1659]
        tunnel: w1639 -> [w1657]
        stop <- w1658 stop-if-true
        n769 = property on="Time Interval" class="DigNum (strict)"() -> ("Value"=w1652:dbl)  [unwired: 2 in, 2 out]
        n770 = property on="Temp. [°C]" class="DigNum (strict)"() -> ("Value"=w1645:dbl)  [unwired: 2 in, 2 out]
        n771 = property on="Mixing RPM" class="DigNum (strict)"() -> ("Value"=w1648:dbl)  [unwired: 2 in, 2 out]
        n772 = for {
          tunnel: w1659 -> [w1676] mode=indexing
          n773 = property class="DigNum (strict)"(reference=w1676) -> (reference out=w1674:refnum<vi>, "Value"=w1673:dbl)  [unwired: 1 in, 1 out]
          n774 = Not Equal?(x=w1673, y=0.0) -> (x != y?=w1675:bool)
          n775 = case shown="True" w1675 {
            tunnel: w1674 -> [_ w1678]
            frame False {
            }
            frame True {
              n776 = property class="DigNum (strict)"(reference=w1678, "NumText.BGColor"=u32 65280 ("Numeric Text.Text Colors:BG Color")) -> ()  [unwired: 1 in, 2 out]
            }
          }
        }
        n777 = for {
          tunnel: w1657 -> [w1669] mode=indexing
          n778 = property class="Str"(reference=w1669) -> (reference out=w1667:refnum<vi>, "Value"=w1666:string)  [unwired: 1 in, 1 out]
          n779 = Not Equal?(x=w1666, y="") -> (x != y?=w1668:bool)
          n780 = case shown="True" w1668 {
            tunnel: w1667 -> [_ w1671]
            frame False {
            }
            frame True {
              n781 = property class="Str"(reference=w1671, "Text.BGColor"=u32 65280 ("Numeric Text.Text Colors:BG Color")) -> ()  [unwired: 1 in, 2 out]
            }
          }
        }
        n782 = Not Equal?(x=w1652, y=30.0) -> (x != y?=w1653:bool)
        n783 = Not Equal?(x=w1645, y=70.0) -> (x != y?=w1646:bool)
        n784 = Not Equal?(x=w1648, y=900.0) -> (x != y?=w1649:bool)
        n785 = case shown="True" w1653 {
          frame False {
          }
          frame True {
            n786 = property on="Time Interval" class="DigNum (strict)"("NumText.BGColor"=u32 65280 ("Numeric Text.Text Colors:BG Color")) -> ()  [unwired: 2 in, 2 out]
          }
        }
        n787 = case shown="True" w1646 {
          frame False {
          }
          frame True {
            n788 = property on="Temp. [°C]" class="DigNum (strict)"("NumText.BGColor"=u32 65280 ("Numeric Text.Text Colors:BG Color")) -> ()  [unwired: 2 in, 2 out]
          }
        }
        n789 = case shown="True" w1649 {
          frame False {
          }
          frame True {
            n790 = property on="Mixing RPM" class="DigNum (strict)"("NumText.BGColor"=u32 65280 ("Numeric Text.Text Colors:BG Color")) -> ()  [unwired: 2 in, 2 out]
          }
        }
        n791 = property on="Loading Delay" class="AbsTime (strict)"() -> ("Value"=w1654:timestamp)  [unwired: 2 in, 2 out]
        n792 = property on="Mixing Time" class="DigNum (strict)"() -> ("Value"=w1642:dbl)  [unwired: 2 in, 2 out]
        n793 = Not Equal?(x=w1654, y=timestamp(-7191 s since 1904-01-01) ("Syrup Preparation Time")) -> (x != y?=w1655:bool)
        n794 = Not Equal?(x=w1642, y=1200.0) -> (x != y?=w1650:bool)
        n795 = case shown="True" w1655 {
          frame False {
          }
          frame True {
            n796 = property on="Loading Delay" class="AbsTime (strict)"("NumText.BGColor"=u32 65280 ("Numeric Text.Text Colors:BG Color")) -> ()  [unwired: 2 in, 2 out]
          }
        }
        n797 = case shown="True" w1650 {
          frame False {
          }
          frame True {
            n798 = property on="Mixing Time" class="DigNum (strict)"("NumText.BGColor"=u32 65280 ("Numeric Text.Text Colors:BG Color")) -> ()  [unwired: 2 in, 2 out]
          }
        }
        n799 = property on="Stop Program" class="Bool (strict)"() -> ("Value"=w1658:bool)  [unwired: 2 in, 2 out]
        n800 = Wait (ms)(milliseconds to wait=u32 1000) -> ()  [unwired: 1 out]
      }
    }
  }
